vi "GIS Printer_Process.vi"(8 "error in":errorcluster, 9 "notifierSync":refnum<notifier>, 10 "TopLevel":refnum<class "TopLevel.lvclass">, 11 "GIS Printer in":refnum<class "GIS Printer.lvclass">) -> (3 "GIS Printer out":refnum<class "GIS Printer.lvclass">)   [LabVIEW 2022 SP3, in "GIS Printer.lvclass"]
uses:
  GIS Printer.lvclass
  TopLevel/TopLevel.lvclass
  Typedefs/PrinterCmdStatus--Enum.ctl
  Typedefs/Command Data.ctl
  Typedefs/API Event Data.ctl
  Typedefs/API Task State.ctl
  Typedefs/API Command Cluster.ctl
  Typedefs/API Command Enum.ctl
  Typedefs/PrinterResponse--Cluster.ctl
  Typedefs/PrinterCommand--Cluster.ctl
  Motor Controller/Motor Controller.lvclass
  AbortProcess.vi
panel:
  in  "C33":bool
  in  "I33 3":bool
  in  "I33 2":bool
  in  "I33 1":bool
  in  "A33":bool
  in  "C22":bool
  in  "A22":bool
  in  "C11":bool
  in  "A11":bool
  in  "C1":bool
  in  "A1":bool
  in  "C2":bool
  in  "A2":bool
  in  "C3":bool
  in  "A3":bool
  in  "C4":bool
  in  "A4":bool
  out "error out":errorcluster
  in  "OK":bool
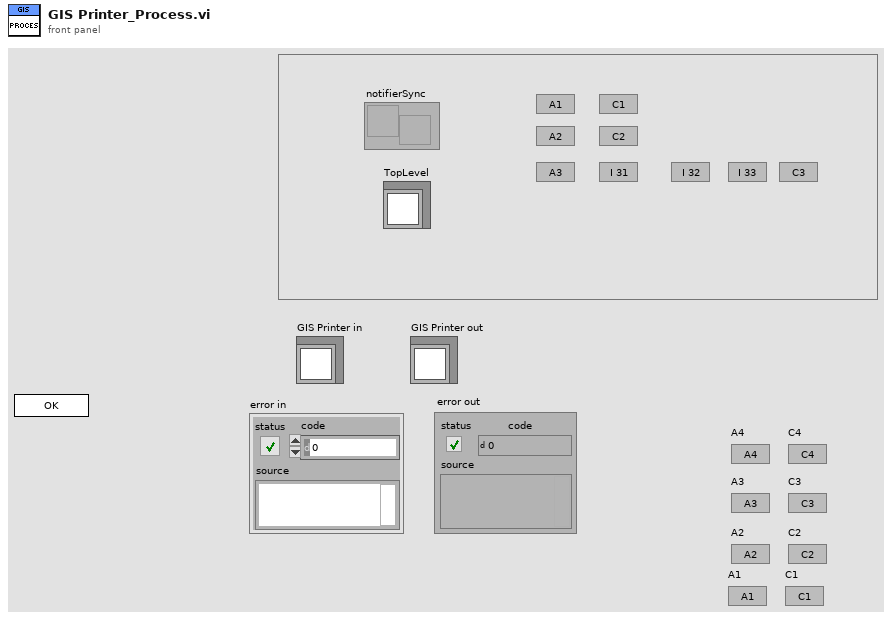
[diagram p1: front panel]
types:
  T1 = cluster{"String":string, "PrinterResponse":refnum<user-event>, "TCP":refnum<k5>, "Open":bool, "TCP 2":refnum<k5>, "Open 2":bool}
  T2 = typedef "GIS Printer.lvclass/PrinterCmdStatus--Enum.ctl" = enum16{"WaitingForAck", "Executing", "Executing Standby", "Completed", "Error"}
  T3 = typedef "GIS Printer.lvclass/Command Data.ctl" = cluster{"PrinterResponse":string, "Cmd Status":T2}
  T4 = typedef "GIS Printer.lvclass/API Event Data.ctl" = cluster{"Task":cluster{"Time Stamp":timestamp, "Timeout (ms)":u32, "Task State":T5, "Task Error":errorcluster, "Task ID":string}, "Command":variant, "Return Value":variant}
  T5 = typedef "GIS Printer.lvclass/API Task State.ctl" = enum16{"Completed", "Errored", "Pending"}
  T6 = typedef "GIS Printer.lvclass/API Command Cluster.ctl" = cluster{"Command":T7, "Arguments":string}
  T7 = typedef "GIS Printer.lvclass/API Command Enum.ctl" = enum16{"Execute Printer Command", "Abort"}
  T8 = enum32{"invalid app kind", "Development System", "Run Time System", "Student Edition", "Embedded LabVIEW", "Evaluation", "Custom"}
  T9 = typedef "GIS Printer.lvclass/PrinterCommand--Cluster.ctl" = cluster{"WaitFor":string, "SentTime":dbl, "PrinterCmdStatus":T2}
  T10 = enum32{"Invalid", "Standard", "Closed", "Hidden", "Minimized", "Maximized"}
  T11 = typedef "GIS Printer.lvclass/PrinterResponse--Cluster.ctl" = cluster{"Command":string, "Response[]":string[], "LastResponse":string, "WaitFor":string}
  T12 = cluster{"Time Stamp":timestamp, "Timeout (ms)":u32, "Task State":T5, "Task Error":errorcluster, "Task ID":string}
  T13 = typedef "GIS Printer.lvclass/PrinterConfiguration--Cluster.ctl" = cluster{"IPAddress":string, "Move Stage on RTP Command?":bool, "Stage Move Position":string, "PH1-Prime Path":path, "PH2-Prime Path":path, "PH3-Prime Path":path, "PH4-Prime Path":path, "PH5-Prime Path":path, "PH6-Prime Path":path, "PrintScriptsFolder":path, "PurgeScriptsFolder":path, "StageScriptsFolder":path, "PH1-HeatOn Path":path, "PH2-HeatOn Path":path, "PH3-HeatOn Path":path, "PH4-HeatOn Path":path, "PH5-HeatOn Path":path, "PH6-HeatOn Path":path, "PH1-HeatOff Path":path, "PH2-HeatOff Path":path, "PH3-HeatOff Path":path, "PH4-HeatOff Path":path, "PH5-HeatOff Path":path, "PH6-HeatOff Path":path}
  T14 = cluster{"Core":cluster{"Current VI Reference":refnum<vi>, "Close Panel on Exit?":bool}, "GIS Printer in":refnum<class "GIS Printer.lvclass">, "Tasks":T4[], "TO":i32, "API Executed Event":refnum<user-event>, "API Return Event":refnum<user-event>, "Task Start ms":u32, "Current Task. Return Value":variant, "TCP":refnum<k5>, "PrinterConfiguration":T13, "CmdMap":map{string, T11}, "CurrentTask":T6, "IDmap":map{string, T9}, "Motor Controller":refnum<class "Motor Controller.lvclass">, "TCP 2":refnum<k5>, "notifierSync":refnum<notifier>}
  T15 = cluster{"Current VI Reference":refnum<vi>, "Close Panel on Exit?":bool}
  T16 = typedef "TopLevel.lvclass/Digilens Config Cluster.ctl" = cluster{"Motion Controller":T17, "IO Config":T18, "PrinterConfiguration":T13, "DAQ Settings":T21}
  T17 = typedef "Motor Controller.lvclass/Motor Controller Config Data.ctl" = cluster{"Motor IP Addresss":string, "Current Position":i32, "Pulse_Per_mm":i32, "PrePrint":dbl[], "Load Position_mm":i32, "Laminate Position_mm":i32}
  T18 = typedef "IO.lvclass/IO Config Data.ctl" = cluster{"DAQDevices":T19[], "DI Channels":T20[], "DO Channels":T20[], "Material Names":string[], "AI Channels":T20[], "AO Channels":T20[]}
  T19 = typedef "IO.lvclass/DCON_DeviceConfig--Cluster.ctl" = cluster{"COM":string, "DeviceName":string, "BaudRate":u32, "Number of Channels":i32, "DeviceAddress":i32, "Enable":bool}
  T20 = typedef "IO.lvclass/Channel Data.ctl" = cluster{"Channel Name":string, "Device Name":string, "Channel No":string}
  T21 = typedef "DAQ.lvclass/TD DAQ Settings--cluster.ctl" = cluster{"Simulate DAQ":bool, "DI Settings":T22[], "AI Settings":T23[], "Relay IONames":string[], "AO IONames":string[], "AO NChan SingleTask":bool}
  T22 = typedef "DAQ.lvclass/TD DI Instrument Settings--cluster.ctl" = cluster{"Disable":bool, "DI TaskName":string, "DI RefreshIntv":i32}
  T23 = typedef "DAQ.lvclass/TD AI Instrument Settings--cluster.ctl" = cluster{"Disable":bool, "AI TaskName":string, "AI InstSettings":T24, "SimAI Ranges":T25}
  T24 = typedef "DAQ.lvclass/TD AI InstSettings--cluster.ctl" = cluster{"DaqRate":dbl, "NumSamples":i32}
  T25 = typedef "DAQ.lvclass/TD SimAI Ranges--cluster.ctl" = cluster{"lo":dbl, "hi":dbl}
  T26 = typedef "GIS Printer.lvclass/UserEvents.ctl" = cluster{"API Incoming Event":refnum<user-event>, "API Executed Event":refnum<user-event>, "API Return Event":refnum<user-event>, "Status Changed Event":refnum<user-event>, "Abort":refnum<user-event>, "stop process":refnum<user-event>, "GISPollStatus":refnum<user-event>, "GISHeadStatus":refnum<user-event>, "Error Event":refnum<user-event>}
  T27 = typedef "TopLevel.lvclass/UserEvents.ctl" = cluster{"API Incoming Event":refnum<user-event>, "API Executed Event":refnum<user-event>, "API Return Event":refnum<user-event>, "Exit Event":refnum<user-event>, "StatusChanged":refnum<user-event>, "DLP GUI Config Changed":refnum<user-event>, "AppEvent":refnum<user-event>, "Login Event":refnum<user-event>}
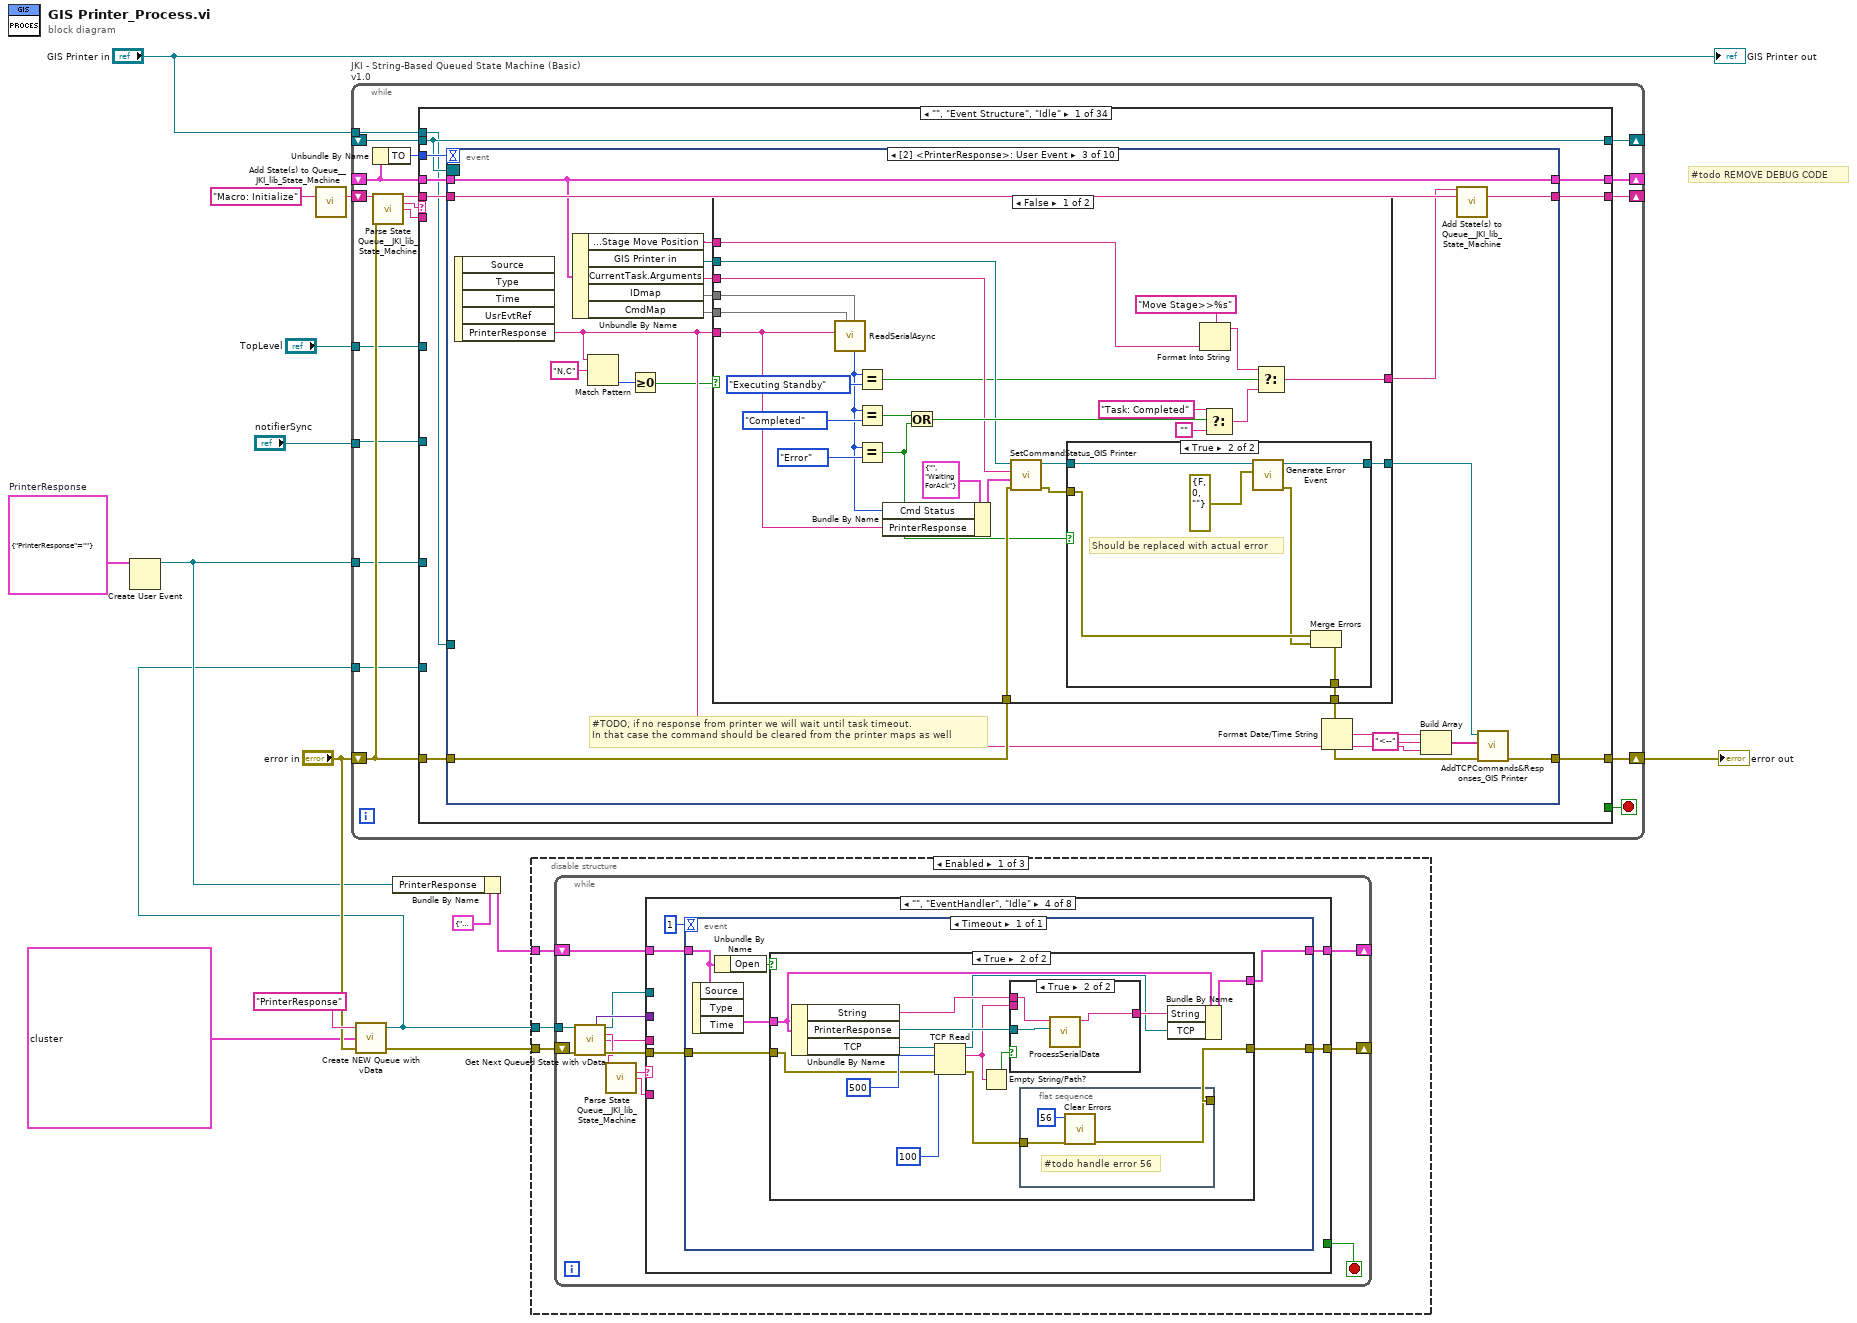
[diagram p0: block diagram]
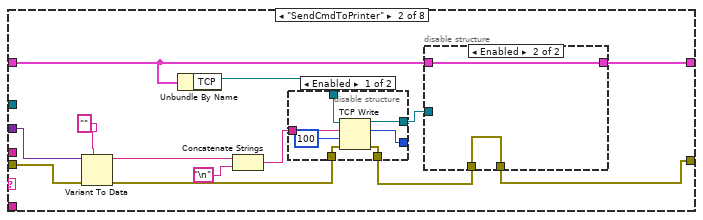
[diagram p3: hidden frame]
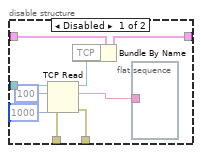
[diagram p4: hidden frame]
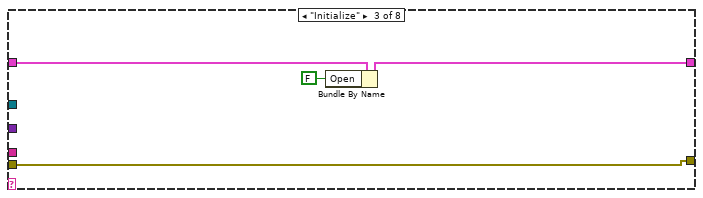
[diagram p6: hidden frame]
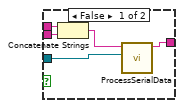
[diagram p8: hidden frame]
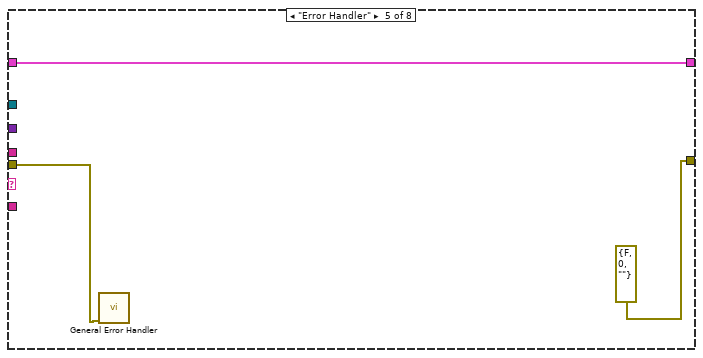
[diagram p9: hidden frame]
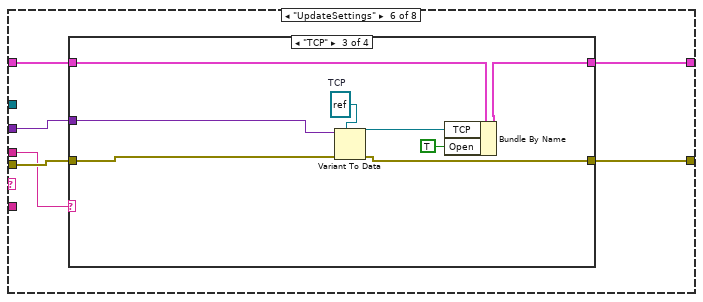
[diagram p10: hidden frame]
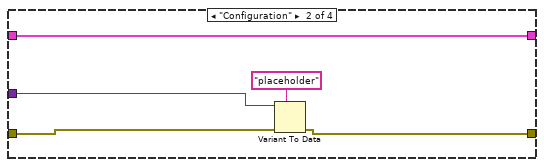
[diagram p12: hidden frame]
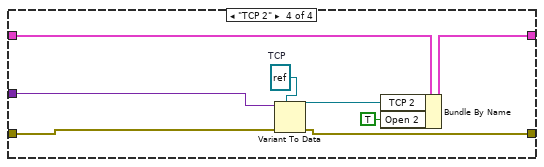
[diagram p13: hidden frame]
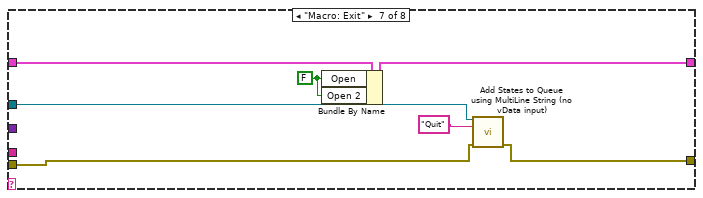
[diagram p14: hidden frame]
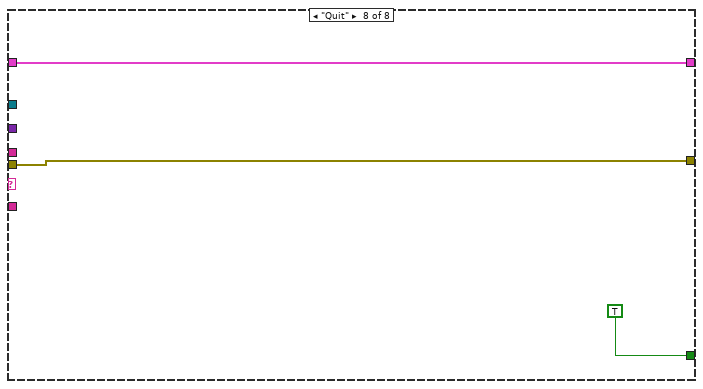
[diagram p15: hidden frame]
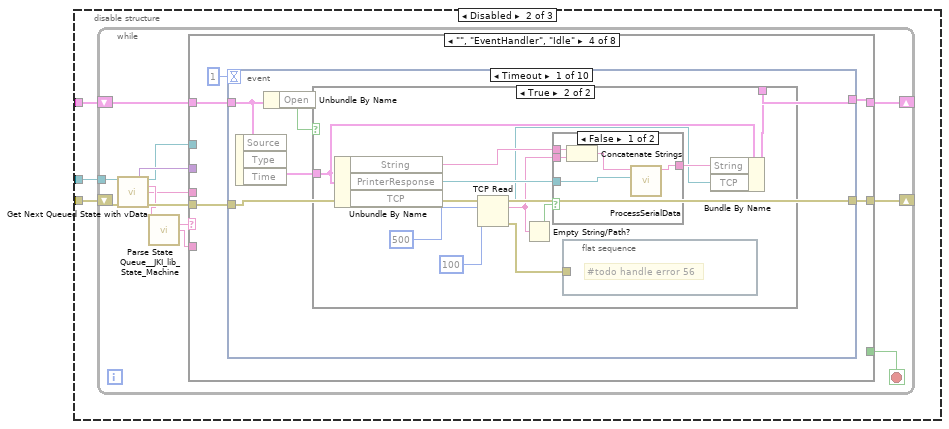
[diagram p16: hidden frame]
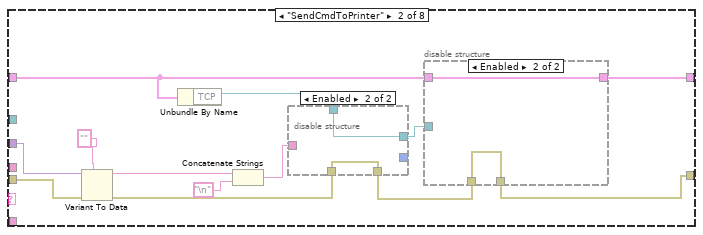
[diagram p18: hidden frame]
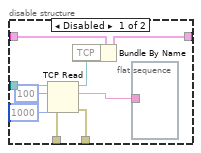
[diagram p19: hidden frame]
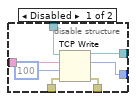
[diagram p20: hidden frame]
diagram:
  w10 = cluster{"PrinterResponse":string} {"PrinterResponse"=""}  # PrinterResponse
  # "#todo REMOVE DEBUG CODE"
  n1 = Create User Event(user event datatype=w10) -> (user event=w3:refnum<user-event>)  [unwired: 1 in, 1 out]
  n2 = call <vilib>:"Add State(s) to Queue__JKI_lib_State_Machine.vi"("State(s) in (\"\")"="Macro: Initialize") -> ("States Out"=w15:string)  [unwired: 14 in]
  n3 = call <vilib>:"Create NEW Queue with vData.vi"("error in (no error)"="error in", "Initial States"=cluster{"state":string, "vData":variant}[] [{"state"="Initialize", "vData"=variant}, {"state"="Idle", "vData"=variant}], "Name (SMQ)"="PrinterResponse") -> ("error out"=w8:errorcluster, "queue out"=w2:refnum<queue>)  [unwired: 1 in]
  n4 = while "JKI - String-Based Queued State Machine (Basic) v1.0" {
    shift-right: [w26] -> _
    shift-left: _ -> [w20]
    shift-right: [w29] -> w12
    shift-left: "error in" -> [w25]
    shift-right: [w28] -> _
    shift-left: w15 -> [w30]
    tunnel: "GIS Printer in" -> [w24]
    shift-right: [w23] -> _
    shift-left: _ -> [w22]
    tunnel: "TopLevel" -> [w19]
    tunnel: w3 -> [w18]
    tunnel: w2 -> [w17]
    tunnel: "notifierSync" -> [w16]
    stop <- w27 stop-if-true
    n5 = Unbundle By Name(w20) -> ("TO"=w21:i32)
    n6 = call <vilib>:"Parse State Queue__JKI_lib_State_Machine.vi"("State Queue"=w30, "Error In (no error)"=w25) -> ("Remaining States"=w32:string, "Current State"=w33:string, "Arguments"=w31:string)  [unwired: 11 in]
    n7 = case shown="\"\", \"Event Structure\", \"Idle\"" w33 {
      selector: w33 -> [_ _ w250 _ _ _ _ _ _ _ _ _ _ _ _ _ _ _ _ _ _ _ _ _ _ _ _ _ _ _ _ _ _ _]
      tunnel: w32 -> [w42 w248 w254 w273 w280 w286 w291 w299 w334 w341 w346 w352 w359 w371 w398 _ w417 w421 w439 w444 w446 _ w504 w519 w534 w542 w559 w570 w589 w606 w622 w642 w667 w705]
      tunnel: w31 -> [_ _ _ _ _ _ _ _ _ _ _ _ w354 w365 _ _ _ _ _ _ _ _ _ _ _ w536 _ _ _ _ _ _ _ _]
      tunnel: w20 -> [w40 w245 w252 w264 w277 w284 w288 w294 _ w336 w343 w350 w357 w367 w395 w400 w415 w419 w436 w443 w447 w454 w503 w520 w524 w541 w560 w567 w586 w605 w620 w640 w664 w702]
      tunnel: [w39 w246 w256 w270 errorcluster {"status"=FALSE, "code"=0, "source"=""} ("error out") w283 w289 w293 w326 w337 w344 w347 w355 w368 w396 w403 w406 w420 w434 w442 w445 w455 w483 w518 w525 w537 w558 w565 w584 w600 w616 w637 w672 w701] -> w29
      tunnel: w25 -> [w38 w246 w255 w270 w276 w283 w289 w292 w325 w338 w344 w348 w356 w369 w396 w403 w405 w420 w426 w441 w445 w461 w494 w518 w525 w539 w558 w568 w587 w604 w615 w636 w671 w700]
      tunnel: [w41 w247 w253 w272 w279 w285 w290 w298 w333 w340 w345 w351 w358 w370 w397 w402 w416 w421 w438 w444 w446 w467 w504 w519 w534 w542 w559 w570 w589 w606 w622 w642 w668 w706] -> w28
      tunnel: [_ _ _ _ _ TRUE _ _ _ _ _ _ _ _ _ _ _ _ _ _ _ _ _ _ _ _ _ _ _ _ _ _ _ _] -> w27
      tunnel: [w37 w245 w252 w271 w277 w284 w288 w294 w332 w336 w343 w350 w357 w367 w395 w400 w415 w419 w436 w443 w447 w459 w499 w520 w524 w541 w560 w569 w588 w605 w620 w640 w665 w699] -> w26
      tunnel: w21 -> [w36 _ _ _ _ _ _ _ _ _ _ _ _ _ _ _ _ _ _ _ _ _ _ _ _ _ _ _ _ _ _ _ _ _]
      tunnel: w24 -> [w34 _ _ _ _ _ _ _ w327 _ _ _ _ _ _ _ _ _ _ _ _ _ _ _ _ _ _ _ _ _ _ w632 w663 _]
      tunnel: [w35 w244 w249 w261 w274 w281 w287 w297 w330 w335 w342 w349 w353 w364 w394 w399 w408 w418 w437 w440 w448 w468 w505 w521 w535 w543 w561 w571 w590 w607 w621 w641 w675 w707] -> w23
      tunnel: w22 -> [w35 w244 w249 w261 w274 w281 w287 w297 w330 w335 w342 w349 w353 w364 w394 w399 w408 w418 _ w440 w448 w468 w505 w521 w535 w543 w561 w571 w590 w607 w621 w641 w675 w707]
      tunnel: w19 -> [_ _ _ _ _ _ _ _ w318 _ _ _ _ _ _ _ _ _ w429 _ _ _ _ _ w522 _ _ _ _ _ _ _ _ _]
      tunnel: w18 -> [_ _ _ _ _ _ _ _ _ _ _ _ _ _ _ _ _ _ w425 _ _ _ _ _ _ _ _ _ _ _ _ _ _ _]
      tunnel: w17 -> [_ _ _ _ _ _ _ _ _ _ _ _ _ _ _ _ w404 _ _ _ _ _ w477 _ _ _ _ w564 w583 _ _ _ _ _]
      tunnel: w16 -> [_ _ _ _ _ _ _ _ w300 _ _ _ _ _ _ _ _ _ _ _ _ _ _ _ _ _ _ _ _ _ _ _ _ _]
      frame "", "Event Structure", "Idle" {
        n8 = event shown="[2] <PrinterResponse>: User Event" {
          selector: w35 -> [_ _ _ _ _ _ _ _ _ _]
          dyn-events: _ -> [_ _ _ _ _ _ _ _ _ _]
          timeout: w36 -> [_ _ _ _ _ _ _ _ _ _]
          tunnel: w42 -> [w51 w56 w76 w119 w124 w132 w138 w142 w150 w227]
          tunnel: [w50 w55 w75 w118 w123 w131 w137 w141 w151 w228] -> w41
          tunnel: w40 -> [w48 w53 w74 w116 w121 w126 w135 w139 w154 w226]
          tunnel: [w49 w54 w63 w117 w122 w130 w136 w140 w153 w220] -> w39
          tunnel: w38 -> [w49 w54 w68 w117 w122 w130 w136 w140 w152 w221]
          tunnel: [w48 w53 w74 w116 w121 w127 w135 w139 w155 w223] -> w37
          tunnel: w34 -> [_ _ _ _ _ _ _ _ w143 _]
          event Timeout {
            n9 = event-data() -> ()  [unwired: 1 in, 1 out]
            n10 = Unbundle By Name(w48) -> ("Tasks"=w47:T4[])
            n11 = Empty Array?(array=w47) -> (empty?=w46:bool)
            n12 = Select(t="", s=w46, f="Task: Check Timeout") -> (s? t:f=w43:string)
            n13 = call <vilib>:"Add State(s) to Queue__JKI_lib_State_Machine.vi"("State(s) in Front (\"\")"=w43, "State(s) in (\"\")"=w51) -> ("States Out"=w50:string)  [unwired: 13 in]
          }
          event User Event {
            n14 = event-data() -> ()  [unwired: 1 in, 5 out]
            n15 = call <vilib>:"Add State(s) to Queue__JKI_lib_State_Machine.vi"("State(s) in Front (\"\")"="API: Abort" ("State(s) in Front (\"\")"), "State(s) in (\"\")"=w56) -> ("States Out"=w55:string)  [unwired: 13 in]
          }
          event User Event {
            # "#TODO, if no response from printer we will wait until task timeout.\nIn that case the command should be cleared from the printer maps as well"
            n16 = event-data() -> ("PrinterResponse"=w61:string)  [unwired: 1 in, 4 out]
            n17 = Unbundle By Name(w74) -> ("PrinterConfiguration.Stage Move Position"=w57:string, "GIS Printer in"=w70:refnum<class "GIS Printer.lvclass">, "CurrentTask.Arguments"=w69:string, "IDmap"=w73:map{string, T9}, "CmdMap"=w72:map{string, T11})
            n18 = Match Pattern(string=w61, regular expression="N,C") -> (offset past match=w59:i32)  [unwired: 1 in, 3 out]
            n19 = Greater Or Equal To 0?(x=w59) -> (x >= 0?=w58:bool)
            n20 = case shown="False" w58 {
              tunnel: w73 -> [w103 _]
              tunnel: w72 -> [w102 _]
              tunnel: [w85 ""] -> w71
              tunnel: w70 -> [w95 w113]
              tunnel: w69 -> [w94 _]
              tunnel: w68 -> [w91 w114]
              tunnel: [w77 w113] -> w65
              tunnel: [w79 w114] -> w64
              tunnel: w61 -> [w90 _]
              tunnel: w57 -> [w84 _]
              frame False {
                n21 = call "ReadSerialAsync.vi"("IDmap"=w103, "CmdMap"=w102, "input Str"=w90) -> ("PrinterCmdStatus"=w88:T2)  [unwired: 5 in, 3 out]
                n22 = Equal?(x=w88, y=PrinterCmdStatus--Enum."Executing Standby") -> (x = y?=w87:bool)
                n23 = Equal?(x=w88, y=PrinterCmdStatus--Enum."Completed") -> (x = y?=w100:bool)
                n24 = Equal?(x=w88, y=PrinterCmdStatus--Enum."Error") -> (x = y?=w81:bool)
                n25 = Bundle By Name(cluster=T3 {"PrinterResponse"="", "Cmd Status"=enum."WaitingForAck"} ("Command Data"), "Cmd Status"=w88, "PrinterResponse"=w90) -> (w92:T3)
                n26 = Or(x=w100, y=w81) -> (x .or. y?=w98:bool)
                n27 = call-dynamic "SetCommandStatus_GIS Printer.vi"("error in (no error)"=w91, "Command Data"=w92, "Command"=w94, "GIS Printer In"=w95) -> ("error out"=w80:errorcluster, "GIS Printer Out"=w78:refnum<class "GIS Printer.lvclass">)  [unwired: 6 in]
                n28 = case shown="True" w81 {
                  tunnel: w80 -> [w105 w108]
                  tunnel: [w105 w107] -> w79
                  tunnel: w78 -> [w104 w110]
                  tunnel: [w104 w109] -> w77
                  frame False {
                  }
                  frame True {
                    # "Should be replaced with actual error"
                    n29 = call-dynamic "Generate Error Event.vi"("Error"=errorcluster {"status"=FALSE, "code"=0, "source"=""}, "GIS Printer in"=w110) -> ("error out"=w106:errorcluster, "GIS Printer out"=w109:refnum<class "GIS Printer.lvclass">)  [unwired: 8 in]
                    n30 = Merge Errors(w108, w106) -> (w107:errorcluster)
                  }
                }
                n31 = Format Into String(format string="Move Stage>>%s" ("t"), w84) -> (resulting string=w82:string)  [unwired: 2 in, 1 out]
                n32 = Select(t="Task: Completed", s=w98, f="") -> (s? t:f=w86:string)
                n33 = Select(t=w82, s=w87, f=w86) -> (s? t:f=w85:string)
              }
              frame True {
                # "NC means good connection\nNZ is bad"
              }
            }
            n34 = Format Date/Time String() -> (date/time string=w67:string)  [unwired: 3 in]
            n35 = Build Array(w67, "<--", w61) -> (w62:string[])
            n36 = call <vilib>:"Add State(s) to Queue__JKI_lib_State_Machine.vi"("State(s) in Front (\"\")"=w71, "State(s) in (\"\")"=w76) -> ("States Out"=w75:string)  [unwired: 13 in]
            n37 = call-dynamic "AddTCPCommands&Responses_GIS Printer.vi"("error in (no error)"=w64, "Command \\ Response"=w62, "GIS Printer In"=w65) -> ("error out"=w63:errorcluster)  [unwired: 7 in, 1 out]
          }
          event "OK": Value Change {
            # "Exit Button Value Change (pressed) Event\n(this executes Macro: Exit to terminate the VI)"
            n38 = event-data() -> ()  [unwired: 1 in, 1 out]
            n39 = call <vilib>:"Add State(s) to Queue__JKI_lib_State_Machine.vi"("State(s) in Front (\"\")"="Macro: Exit", "State(s) in (\"\")"=w119) -> ("States Out"=w118:string)  [unwired: 13 in]
          }
          event User Event {
            # "Exit Button Value Change (pressed) Event\n(this executes Macro: Exit to terminate the VI)"
            n40 = event-data() -> ()  [unwired: 1 in, 5 out]
            n41 = disable-structure shown="Disabled" {
              disable-tunnel: ["Macro: Exit" _] -> w120
              frame Disabled {
              }
              frame Enabled {
              }
            }
            n42 = call <vilib>:"Add State(s) to Queue__JKI_lib_State_Machine.vi"("State(s) in Front (\"\")"=w120, "State(s) in (\"\")"=w124) -> ("States Out"=w123:string)  [unwired: 13 in]
          }
          event User Event {
            n43 = event-data() -> ("Command"=w129:string, "Data"=w128:variant)  [unwired: 1 in, 4 out]
            n44 = case shown="Default" w129 {
              tunnel: w128 -> [_]
              tunnel: w126 -> [w133]
              tunnel: [w133] -> w127
              frame Default {
              }
            }
            n45 = call <vilib>:"Add State(s) to Queue__JKI_lib_State_Machine.vi"("State(s) in (\"\")"=w132) -> ("States Out"=w131:string)  [unwired: 14 in]
          }
          event User Event {
            # "Exit Button Value Change (pressed) Event\n(this executes Macro: Exit to terminate the VI)"
            n46 = event-data() -> ()  [unwired: 1 in, 5 out]
            n47 = call <vilib>:"Add State(s) to Queue__JKI_lib_State_Machine.vi"("State(s) in Front (\"\")"="Macro: Exit", "State(s) in (\"\")"=w138) -> ("States Out"=w137:string)  [unwired: 13 in]
          }
          event Panel Close? {
            # "Close Panel button (pressed) Event\n(this executes Macro: Exit to terminate the VI)"
            n48 = event-data() -> ()  [unwired: 1 in, 1 out]
            n49 = event-data() -> ()  [unwired: 2 in, 1 out]
            n50 = call <vilib>:"Add State(s) to Queue__JKI_lib_State_Machine.vi"("State(s) in (\"\")"=w142) -> ("States Out"=w141:string)  [unwired: 14 in]
          }
          event User Event {
            n51 = event-data() -> ("Task"=w158:T12, "Command"=w157:variant)  [unwired: 1 in, 4 out]
            n52 = Bundle By Name(cluster=T4 {"Task"={"Time Stamp"=timestamp(0 s since 1904-01-01), "Timeout (ms)"=0, "Task State"=enum."Completed", "Task Error"={"status"=FALSE, "code"=0, "source"=""}, "Task ID"=""}, "Command"=variant, "Return Value"=variant} ("API Event Data"), "Task"=w158, "Command"=w157) -> (w148:T4)
            n53 = Unbundle By Name(w154) -> ("Tasks"=w156:T4[])
            n54 = Unbundle By Name(w148) -> ("Task.Task ID"=w147:string)
            n55 = Empty Array?(array=w156) -> (empty?=w145:bool)
            n56 = Equal?(x=w147, y="AbortPrint") -> (x = y?=w144:bool)
            n57 = case shown="True" w144 {
              tunnel: w156 -> [w168 _]
              tunnel: [w167 w207] -> w155
              tunnel: w154 -> [w166 w207]
              tunnel: [w165 w196] -> w153
              tunnel: w152 -> [w164 w198]
              tunnel: [w163 w199] -> w149
              tunnel: w148 -> [w162 w200]
              tunnel: w145 -> [w161 _]
              tunnel: w143 -> [w160 _]
              frame False {
                n58 = case shown="True" w161 {
                  tunnel: w168 -> [w189 w195]
                  tunnel: w162 -> [w188 w194]
                  tunnel: w166 -> [w187 w193]
                  tunnel: [w185 w191] -> w167
                  tunnel: w162 -> [w184 _]
                  tunnel: w164 -> [w169 w190]
                  tunnel: [w180 w190] -> w165
                  tunnel: [w177 _] -> w163
                  tunnel: w160 -> [w172 _]
                  frame True {
                    n59 = Unbundle By Name(w184) -> ("Command"=w183:variant)
                    n60 = call-dynamic "SetPrinterBusy_Status_GIS Printer.vi"("error in (no error)"=w169, "Printer Busy?"=TRUE, "GIS Printer In"=w172) -> ("error out"=w170:errorcluster)  [unwired: 7 in, 1 out]
                    n61 = Build Array (concatenate)(w189, w188) -> (w186:T4[])
                    n62 = Variant To Data(error in=w170, type=T6 {"Command"=enum."Execute Printer Command", "Arguments"=""} ("API Command Cluster"), Variant=w183) -> (data=w173:T6, error out=w181:errorcluster)
                    n63 = Tick Count (ms)() -> (millisecond timer value=w175:u32)
                    n64 = Unbundle By Name(w173) -> ("Command"=w178:T7, "Arguments"=w176:string)
                    n65 = Bundle By Name(cluster=w187, "TO"=100, "Tasks"=w186, "Task Start ms"=w175, "CurrentTask"=w173) -> (w185:T14)
                    n66 = Format Into String(format string="API: %s>>%s", error in=w181, w178, w176) -> (resulting string=w177:string, error out=w180:errorcluster)  [unwired: 1 in]
                  }
                  frame False {
                    n67 = Build Array (concatenate)(w195, w194) -> (w192:T4[])
                    n68 = Bundle By Name(cluster=w193, "Tasks"=w192) -> (w191:T14)
                  }
                }
              }
              frame True {
                # "Abort should not send a task complete"
                n69 = Unbundle By Name(w200) -> ("Command"=w206:variant)
                n70 = Variant To Data(error in=w198, type=T6 {"Command"=enum."Execute Printer Command", "Arguments"=""} ("API Command Cluster"), Variant=w206) -> (data=w201:T6, error out=w197:errorcluster)
                n71 = Unbundle By Name(w201) -> ("Command"=w203:T7, "Arguments"=w202:string)
                n72 = Format Into String(format string="API: %s>>%s", error in=w197, w203, w202) -> (resulting string=w199:string, error out=w196:errorcluster)  [unwired: 1 in]
              }
            }
            n73 = call <vilib>:"Add State(s) to Queue__JKI_lib_State_Machine.vi"("State(s) in Front (\"\")"=w149, "State(s) in (\"\")"=w150) -> ("States Out"=w151:string)  [unwired: 13 in]
          }
          event User Event {
            n74 = event-data() -> ("Task"=w214:T12, "Command"=w218:variant, "Return Value"=w217:variant)  [unwired: 1 in, 4 out]
            n75 = Unbundle By Name(w226) -> ("API Return Event"=w211:refnum<user-event>, "Tasks"=w225:T4[])
            n76 = Bundle By Name(cluster=T4 {"Task"={"Time Stamp"=timestamp(0 s since 1904-01-01), "Timeout (ms)"=0, "Task State"=enum."Completed", "Task Error"={"status"=FALSE, "code"=0, "source"=""}, "Task ID"=""}, "Command"=variant, "Return Value"=variant} ("API Event Data"), "Task"=w214, "Command"=w218, "Return Value"=w217) -> (w216:T4)
            n77 = Delete From Array(array=w225, index=0) -> (deleted portion=w215:T4, array with subset deleted=w222:T4[])  [unwired: 1 in]
            n78 = Unbundle By Name(w215) -> ("Task.Task ID"=w213:string)
            n79 = Unbundle By Name(w214) -> ("Task ID"=w212:string, "Task State"=w209:T5)
            n80 = Equal?(x=w213, y=w212) -> (x = y?=w210:bool)
            n81 = case shown="True" w210 {
              tunnel: w226 -> [w230 w243]
              tunnel: [w230 w242] -> w223
              tunnel: w222 -> [_ w241]
              tunnel: w211 -> [_ w240]
              tunnel: w221 -> [w229 w237]
              tunnel: [w229 w238] -> w220
              tunnel: w216 -> [_ w239]
              tunnel: w209 -> [_ w236]
              tunnel: [_ w231] -> w208
              frame False {
              }
              frame True {
                n82 = Equal?(x=w236, y=API_Task_State."Errored") -> (x = y?=w234:bool)
                n83 = Select(t="Task: Remove on Error", s=w234, f="Task: Check Pending") -> (s? t:f=w231:string)
                n84 = Bundle By Name(cluster=w243, "Tasks"=w241) -> (w242:T14)
                n85 = Generate User Event(user event=w240, event data cluster=w239, error in=w237) -> (error out=w238:errorcluster)  [unwired: 1 in, 1 out]
              }
            }
            n86 = call <vilib>:"Add State(s) to Queue__JKI_lib_State_Machine.vi"("State(s) in Front (\"\")"=w208, "State(s) in (\"\")"=w227) -> ("States Out"=w228:string)  [unwired: 13 in]
          }
        }
      }
      frame "---------- Core ----------" {
        n87 = call <vilib>:"Add State(s) to Queue__JKI_lib_State_Machine.vi"("State(s) in (\"\")"=w248) -> ("States Out"=w247:string)  [unwired: 14 in]
      }
      frame Default {
        w259 = 42 items=["No error", "Argument error", "Memory is full", "Out of zone", "End of file", "File already open", "Generic file I/O error", "File not found", "File permission error", "Disk is full", "Duplicate path", "Too many files open", "System feature not enabled", "Resource file not found", "Cannot add resource", "Resource not found", "Image not found", "Image memory error", "Pen does not exist", "Config type invalid", "Config token not found", "Config parse error", "Config memory error", "Bad external code format", "Bad external code offset", "External code not present", "Null window", "Destroy window error", "Null menu", "Print aborted", "Bad print record", "Print driver error", "Windows error during printing", "Memory error during printing", "Print dialog error", "Generic print error", "Invalid device refnum", "Device not found", "Device parameter error", "Device unit error", "Cannot open device", "Device call aborted", "Generic error", "Cancelled by user", "Object ID too low", "Object ID too high", "Object not in heap", "Unknown heap", "Unknown object (invalid DefProc)", "Unknown object (DefProc not in table)", "Message out of range", "Invalid (null) method", "Unknown message", "Manager call not supported", "Bad address", "Network operation in progress", "Network operation timed out", "Connection is busy", "Network attribute not supported", "Network error", "Address in use", "System out of memory", "Connection aborted", "Connection refused", "Not connected", "Already connected", "Connection closed", "Initialization error (interapplication manager)", "Bad occurrence", "Wait on unbound occurrence handler", "Occurrence queue overflow", "Datalog type conflict", "Unused", "Unrecognized type (interapplication manager)", "Memory corrupt", "Failed to make temporary DLL", "Old CIN version", "Drag socket not found", "Failed to load drop-object", "Failed to register OLE object", "Failed to release OLE object", "Format specifier type mismatch", "Unknown format specifier", "Too few format specifiers", "Too many format specifiers", "Scan failed", "Newer CIN version", "Error converting to variant", "Runtime menu error", "Password tampered", "Variant attribute not found", "Incompatible variant data type", "Event data is not available", "Event Store is not present", "Occurrence is not found", "Event Queue is not created", "Event info is not available", "Refnum passed is NULL", "Error retrieving Class GUID", "Error retrieving CoClass GUID", "Error retrieving TypeLib GUID.", "Bad built application magic bytes.", "Specific driver is different from the specific driver associated with the Logical Name.", "There is no session opened to the class driver.", "Max Error", "MAX - Error with config objects", "MAX - Error loading configuration", "MAX - Group not supported"]
        # "Current State"
        # "Handle mistyped state name (developer tool)"
        n88 = Format Into String(format string="Software Exception: Unhandled State \"%s\"." ("message"), error in=w255, w250) -> (resulting string=w258:string, error out=w257:errorcluster)  [unwired: 1 in]
        n89 = call <vilib>:"Error Cluster From Error Code.vi"("show call chain? (False)"=TRUE, "error in (no error)"=w257, "error message (\"\")"=w258, "error code (0)"=w259) -> ("error out"=w256:errorcluster)  [unwired: 5 in]
        n90 = call <vilib>:"Add State(s) to Queue__JKI_lib_State_Machine.vi"("State(s) in (\"\")"=w254) -> ("States Out"=w253:string)  [unwired: 14 in]
      }
      frame "Initialize Core Data" {
        # "originally closed?"
        # "exe?"
        # "If panel starts closed or is an EXE, then close it when we exit"
        n91 = property class="VI"() -> ("Front Panel.Open"=w269:bool)  [unwired: 2 in, 2 out]
        n92 = property class="App"() -> ("App.Kind"=w268:T8)  [unwired: 2 in, 2 out]
        n93 = control-ref of="Current VI Reference"() -> (w262:refnum<vi>)
        n94 = Not(x=w269) -> (.not. x?=w266:bool)
        n95 = Equal?(x=w268, y=T8."Run Time System" ("Application:Kind")) -> (x = y?=w265:bool)
        n96 = Or(x=w266, y=w265) -> (x .or. y?=w263:bool)
        n97 = Bundle By Name(cluster=w264, "Core.Current VI Reference"=w262, "Core.Close Panel on Exit?"=w263) -> (w271:T14)
        n98 = call <vilib>:"Add State(s) to Queue__JKI_lib_State_Machine.vi"("State(s) in (\"\")"=w273) -> ("States Out"=w272:string)  [unwired: 14 in]
      }
      frame "Error Handler" {
        # "Unhandled Error -- Display it"
        # "Clear error"
        n99 = call <vilib>:"General Error Handler.vi"("error in (no error)"=w276) -> ()  [unwired: 10 in, 5 out]
        n100 = call <vilib>:"Add State(s) to Queue__JKI_lib_State_Machine.vi"("State(s) in Front (\"\")"="/* Post Error States", "State(s) in (\"\")"=w280) -> ("States Out"=w279:string)  [unwired: 13 in]
      }
      frame "Exit" {
        n101 = call <vilib>:"Add State(s) to Queue__JKI_lib_State_Machine.vi"("State(s) in (\"\")"=w286) -> ("States Out"=w285:string)  [unwired: 14 in]
      }
      frame "---------- Data ----------" {
        n102 = call <vilib>:"Add State(s) to Queue__JKI_lib_State_Machine.vi"("State(s) in (\"\")"=w291) -> ("States Out"=w290:string)  [unwired: 14 in]
      }
      frame "Process: Sync" {
        n103 = Unbundle By Name(w294) -> ("notifierSync"=w296:refnum<notifier>)
        n104 = Send Notification(notification=TRUE, notifier=w296, error in (no error)=w292) -> (error out=w293:errorcluster)  [unwired: 1 out]
        n105 = call <vilib>:"Add State(s) to Queue__JKI_lib_State_Machine.vi"("State(s) in (\"\")"=w299) -> ("States Out"=w298:string)  [unwired: 14 in]
      }
      frame "Data: Initialize" {
        w301 = refnum<k5> refnum  # TCP 2
        w304 = refnum<class "Motor Controller.lvclass"> refnum  # Motor Controller
        w305 = map{string, T9} {}  # IDmap
        w310 = map{string, T11} {}  # CmdMap
        w311 = T11 {"Command"="", "Response[]"=[], "LastResponse"="", "WaitFor"=""}  # Response
        w312 = T6 {"Command"=enum."Execute Printer Command", "Arguments"=""}  # CurrentTask
        w319 = refnum<k5> refnum  # TCP
        w320 = variant  # Current Task. Return Value
        w322 = u32 0  # Task Start ms
        w328 = 100  # TO
        w329 = T4[] []  # Tasks
        w331 = T15 {"Current VI Reference"=refnum, "Close Panel on Exit?"=FALSE}  # Core
        n106 = property class="TopLevel.lvclass"(reference=w318) -> ("Methods:Accessors:Digilens Config"=w317:T16, "Methods:Accessors:Motor Controller"=w303:refnum<class "Motor Controller.lvclass">)  [unwired: 1 in, 2 out]
        n107 = Unbundle By Name(w317) -> ("PrinterConfiguration"=w316:T13)
        n108 = Coerce To Type(0:w303, 1:w304) -> (2:w302:refnum<class "Motor Controller.lvclass">)
        n109 = node("Commands" ("key"), T9 {"WaitFor"="", "SentTime"=0.0, "PrinterCmdStatus"=enum."WaitingForAck"} ("Cluster")) -> (w308:map{string, T9})
        n110 = Coerce To Type(0:w308, 1:w305) -> (2:w307:map{string, T9})
        n111 = call-dynamic "GetEvents_GIS Printer.vi"("error in (no error)"=w325, "TopLevel in"=w327) -> ("error out"=w326:errorcluster, "UserEvents"=w324:T26)  [unwired: 7 in, 1 out]
        n112 = Unbundle By Name(w324) -> ("API Executed Event"=w323:refnum<user-event>, "API Return Event"=w321:refnum<user-event>)
        n113 = node("CmdID" ("key"), w311) -> (w314:map{string, T11})
        n114 = Coerce To Type(0:w314, 1:w310) -> (2:w313:map{string, T11})
        n115 = call <vilib>:"Add State(s) to Queue__JKI_lib_State_Machine.vi"("State(s) in (\"\")"=w334) -> ("States Out"=w333:string)  [unwired: 14 in]
        n116 = Bundle("Core"=w331, "GIS Printer in"=w327, "Tasks"=w329, "TO"=w328, "API Executed Event"=w323, "API Return Event"=w321, "Task Start ms"=w322, "Current Task. Return Value"=w320, "TCP"=w319, "PrinterConfiguration"=w316, "CmdMap"=w313, "CurrentTask"=w312, "IDmap"=w307, "Motor Controller"=w302, "TCP 2"=w301, "notifierSync"=w300) -> (w332:T14)  [unwired: 1 in]
      }
      frame "Data: Cleanup" {
        n117 = Unbundle By Name(w336) -> ("Core.Current VI Reference"=w339:refnum<vi>)
        n118 = Close Reference(reference=w339, error in (no error)=w338) -> (error out=w337:errorcluster)
        n119 = call <vilib>:"Add State(s) to Queue__JKI_lib_State_Machine.vi"("State(s) in (\"\")"=w341) -> ("States Out"=w340:string)  [unwired: 14 in]
      }
      frame "---------- UI ----------" {
        n120 = call <vilib>:"Add State(s) to Queue__JKI_lib_State_Machine.vi"("State(s) in (\"\")"=w346) -> ("States Out"=w345:string)  [unwired: 14 in]
      }
      frame "UI: Initialize" {
        n121 = call <userlib>:"Fit VI window to Largest Dec__ogtk.vi"("error in (no error)"=w348) -> ("error out"=w347:errorcluster)  [unwired: 5 in, 1 out]
        n122 = call <vilib>:"Add State(s) to Queue__JKI_lib_State_Machine.vi"("State(s) in (\"\")"=w352) -> ("States Out"=w351:string)  [unwired: 14 in]
      }
      frame "UI: Cursor Set" {
        # "Argument"
        n123 = case shown="\"Idle\", Default" w354 {
          tunnel: w356 -> [w361 w363]
          tunnel: [w360 w362] -> w355
          frame "Idle", Default {
            n124 = call <vilib>:"Unset Busy.vi"("error in (no error)"=w361) -> ("error out"=w360:errorcluster)  [unwired: 10 in]
          }
          frame "Busy" {
            n125 = call <vilib>:"Set Busy.vi"("error in (no error)"=w363) -> ("error out"=w362:errorcluster)  [unwired: 9 in, 1 out]
          }
        }
        n126 = call <vilib>:"Add State(s) to Queue__JKI_lib_State_Machine.vi"("State(s) in (\"\")"=w359) -> ("States Out"=w358:string)  [unwired: 14 in]
      }
      frame "UI: Front Panel State" {
        # "Argument"
        n127 = Unbundle By Name(w367) -> ("Core.Current VI Reference"=w366:refnum<vi>)
        n128 = case shown="\"Open\", Default" w365 {
          tunnel: w369 -> [w375 w388]
          tunnel: [w377 w389] -> w368
          tunnel: w366 -> [w376 w386]
          frame "Open", Default {
            n129 = property class="VI"(reference=w376, error in=w375) -> (reference out=w373:refnum<vi>, error out=w374:errorcluster, "Front Panel.Open"=w372:bool)
            n130 = case shown="False" w372 {
              tunnel: [w380 w383] -> w377
              tunnel: w374 -> [w379 w383]
              tunnel: w373 -> [w378 _]
              frame False {
                n131 = invoke class="VI" method="FP.Open"(reference=w378, error in=w379, "Activate"=TRUE, "State"=T10."Standard") -> (error out=w380:errorcluster)  [unwired: 1 in, 4 out]
              }
              frame True {
              }
            }
          }
          frame "Close" {
            n132 = property class="VI"(reference=w386, error in=w388) -> (reference out=w385:refnum<vi>, error out=w387:errorcluster, "Front Panel.Open"=w384:bool)
            n133 = case shown="True" w384 {
              tunnel: [w390 w393] -> w389
              tunnel: w387 -> [w390 w392]
              tunnel: w385 -> [_ w391]
              frame False {
              }
              frame True {
                n134 = invoke class="VI" method="FP.Close"(reference=w391, error in=w392) -> (error out=w393:errorcluster)  [unwired: 1 in, 2 out]
              }
            }
          }
        }
        n135 = call <vilib>:"Add State(s) to Queue__JKI_lib_State_Machine.vi"("State(s) in (\"\")"=w371) -> ("States Out"=w370:string)  [unwired: 14 in]
      }
      frame "---------- Macro ----------" {
        n136 = call <vilib>:"Add State(s) to Queue__JKI_lib_State_Machine.vi"("State(s) in (\"\")"=w398) -> ("States Out"=w397:string)  [unwired: 14 in]
      }
      frame "Macro: Initialize" {
        w401 = "Data: Initialize\nInitialize Core Data\nUI: Initialize\nAction: Open Connection\nAction: Open Connection 2\n/*Action: Launch Abort Process\nEvents: Register Events\nProcess: Sync\n/*UI: Front Panel State >> Open"  # Data: Initialize Initialize Core Data UI: Initialize Action: Open Connection Action: Open Connection 2 /*Action: Launch Abort Process Events: Register Events Process: Sync /*UI: Front Panel State >> Open
        n137 = call <vilib>:"Add State(s) to Queue__JKI_lib_State_Machine.vi"("State(s) in (\"\")"=w401) -> ("States Out"=w402:string)  [unwired: 14 in]
      }
      frame "Macro: Exit" {
        n138 = call <vilib>:"Add States to Queue using MultiLine String (no vData input).vi"("queue in"=w404, "states in"="Macro: Exit", "error in"=w405) -> ("error out"=w406:errorcluster)  [unwired: 10 in, 2 out]
        n139 = Unbundle By Name(w415) -> ("Core.Close Panel on Exit?"=w414:bool)
        n140 = Select(t="UI: Front Panel State >> Close", s=w414, f="") -> (s? t:f=w411:string)
        n141 = call <vilib>:"Add State(s) to Queue__JKI_lib_State_Machine.vi"("State(s) in (\"\")"=w411, "State(s) at Back (\"\")"="Data: Cleanup\nEvents: Unregister Events\nAction: Close Connection\nExit") -> ("States Out"=w409:string)  [unwired: 13 in]
        n142 = call <vilib>:"Add State(s) to Queue__JKI_lib_State_Machine.vi"("State(s) in Front (\"\")"=w409, "State(s) in (\"\")"=w417) -> ("States Out"=w416:string)  [unwired: 13 in]
      }
      frame "---------- Events ----------" {
      }
      frame "Events: Register Events" {
        n143 = call-dynamic "GetEvents_TopLevel.vi"("error in (no error)"=w426, "TopLevel in"=w429) -> ("error out"=w427:errorcluster, "UserEvents"=w430:T27)  [unwired: 7 in, 1 out]
        n144 = Unbundle By Name(w430) -> ("Exit Event"=w428:refnum<user-event>, "AppEvent"=w422:refnum<user-event>)
        n145 = Unbundle By Name(w436) -> ("GIS Printer in"=w435:refnum<class "GIS Printer.lvclass">)
        n146 = call-dynamic "GetEvents_GIS Printer.vi"("error in (no error)"=w427, "TopLevel in"=w435) -> ("error out"=w434:errorcluster, "UserEvents"=w433:T26)  [unwired: 7 in, 1 out]
        n147 = Unbundle By Name(w433) -> ("API Incoming Event"=w432:refnum<user-event>, "API Executed Event"=w431:refnum<user-event>, "Abort"=w424:refnum<user-event>, "stop process"=w423:refnum<user-event>)
        n148 = register-events(w432, w431, w428, w425, w424, w423, w422) -> (reference out=w437:refnum<event-registration>)  [unwired: 2 in, 1 out]
        n149 = call <vilib>:"Add State(s) to Queue__JKI_lib_State_Machine.vi"("State(s) in (\"\")"=w439) -> ("States Out"=w438:string)  [unwired: 14 in]
      }
      frame "Events: Unregister Events" {
        n150 = Unregister For Events(event registration refnum=w440, error in=w441) -> (error out=w442:errorcluster)
      }
      frame "---------- API ----------" {
      }
      frame "API: Abort" {
        n151 = Unbundle By Name(w454) -> ("IDmap"=w451:map{string, T9}, "CmdMap"=w452:map{string, T11}, "TCP 2"=w465:refnum<k5>, "GIS Printer in"=w453:refnum<class "GIS Printer.lvclass">)
        n152 = Concatenate Strings("P,A" ("string"), "\n") -> (w464:string)
        n153 = TCP Write(connection ID=w465, data in=w464, error in (no error)=w461, 9:100 ("timeout ms (25000)")) -> (connection ID out=w458:refnum<k5>, error out=w456:errorcluster)  [unwired: 1 out]
        n154 = call-dynamic "SetPrinterBusy_Status_GIS Printer.vi"("error in (no error)"=w456, "Printer Busy?"=FALSE, "GIS Printer In"=w453) -> ("error out"=w455:errorcluster)  [unwired: 7 in, 1 out]
        n155 = for {
          tunnel: w452 -> [w476] mode=indexing
          shift-right: [w473] -> w449
          shift-left: w452 -> [w474]
          n156 = Unbundle By Name(w476) -> ("key"=w475:string)
          n157 = Remove From Map(10:w475, 11:w474) -> (3:w473:map{string, T11})  [unwired: 2 out]
        }
        n158 = for {
          tunnel: w451 -> [w472] mode=indexing
          shift-right: [w469] -> w450
          shift-left: w451 -> [w470]
          n159 = Unbundle By Name(w472) -> ("key"=w471:string)
          n160 = Remove From Map(10:w471, 11:w470) -> (3:w469:map{string, T9})  [unwired: 2 out]
        }
        n161 = call <vilib>:"Add State(s) to Queue__JKI_lib_State_Machine.vi"("State(s) in Front (\"\")"="/*Task: Remove on Error\nAction: Open Connection 2" ("State(s) in Front (\"\")")) -> ("States Out"=w467:string)  [unwired: 14 in]
        n162 = Bundle By Name(cluster=w454, "TCP 2"=w458, "IDmap"=w450, "CmdMap"=w449) -> (w459:T14)
      }
      frame "API: Execute Printer Command" {
        n163 = Unbundle By Name(w503) -> ("IDmap"=w496:map{string, T9}, "CurrentTask"=w501:T6, "TCP"=w498:refnum<k5>, "GIS Printer in"=w488:refnum<class "GIS Printer.lvclass">)
        n164 = Variant To Data(error in=w494, type=T6 {"Command"=enum."Execute Printer Command", "Arguments"=""} ("API Command Cluster"), Variant=w501) -> (data=w500:T6, error out=w495:errorcluster)
        n165 = Unbundle By Name(w500) -> ("Arguments"=w479:string)
        n166 = disable-structure shown="Enabled" {
          disable-tunnel: w498 -> [w511 w517]
          disable-tunnel: [w510 w517] -> w497
          disable-tunnel: w495 -> [w508 w514]
          disable-tunnel: w479 -> [w507 w515]
          disable-tunnel: [w506 w513] -> w486
          disable-tunnel: w477 -> [_ w512]
          frame Disabled {
            n167 = TCP Write(connection ID=w511, data in=w507, error in (no error)=w508, 9:100 ("timeout ms (25000)")) -> (connection ID out=w510:refnum<k5>, error out=w506:errorcluster)  [unwired: 1 out]
          }
          frame Enabled {
            n168 = call <vilib>:"Add State to Queue with vData.vi"("queue in"=w512, "state in"="SendCmdToPrinter", "vData (\"\")"=w515, "error in"=w514) -> ("error out"=w513:errorcluster)  [unwired: 8 in, 3 out]
          }
        }
        n169 = Get Date/Time In Seconds() -> (seconds since 1Jan1904=w482:timestamp)
        n170 = To Double Precision Float(number=w482) -> (double precision float=w491:dbl)
        n171 = Bundle By Name(cluster=T9 {"WaitFor"="", "SentTime"=0.0, "PrinterCmdStatus"=enum."WaitingForAck"} ("value"), "WaitFor"=w479, "SentTime"=w491, "PrinterCmdStatus"=PrinterCmdStatus--Enum."WaitingForAck") -> (w490:T9)
        n172 = Format Date/Time String(seconds (now)=w482) -> (date/time string=w481:string)  [unwired: 2 in]
        n173 = call-dynamic "SetCommandStatus_GIS Printer.vi"("error in (no error)"=w486, "Command Data"=T3 {"PrinterResponse"="", "Cmd Status"=enum."WaitingForAck"}, "Command"=w479, "GIS Printer In"=w488) -> ("error out"=w484:errorcluster, "GIS Printer Out"=w485:refnum<class "GIS Printer.lvclass">)  [unwired: 6 in]
        n174 = Insert Into Map(map in=w496, key=w479, value=w490) -> (map out=w493:map{string, T9})  [unwired: 2 out]
        n175 = Build Array(w481, "-->", w479) -> (w478:string[])
        n176 = Bundle By Name(cluster=w503, "IDmap"=w493, "TCP"=w497) -> (w499:T14)
        n177 = call-dynamic "AddTCPCommands&Responses_GIS Printer.vi"("error in (no error)"=w484, "Command \\ Response"=w478, "GIS Printer In"=w485) -> ("error out"=w483:errorcluster)  [unwired: 7 in, 1 out]
      }
      frame "---------- Action ----------" {
      }
      frame "Action: Launch Abort Process" {
        n178 = Unbundle By Name(w524) -> ("GIS Printer in"=w523:refnum<class "GIS Printer.lvclass">)
        n179 = vi-ref "GIS Printer.lvclass:AbortProcess.vi"() -> (w533:refnum<vi>)
        n180 = property class="VI"(reference=w533) -> ("Name"=w532:string)  [unwired: 1 in, 2 out]
        n181 = Open VI Reference(type specifier VI Refnum (for type only)=refnum<vi> refnum, vi path=w532, options=128, error in (no error)=w525) -> (vi reference=w529:refnum<vi>, error out=w528:errorcluster)  [unwired: 2 in]
        n182 = call-by-ref "Start Asynchronous Call"(reference=w529, error in=w528, 8:"error in (no error)"=w528, "TopLevel"=w522, "GIS Printer in"=w523) -> (reference out=w527:refnum<vi>, error out=w526:errorcluster)  [unwired: 7 in, 2 out]
        n183 = Close Reference(reference=w527, error in (no error)=w526) -> ()  [unwired: 1 out]
      }
      frame "Move Stage" {
        n184 = Unbundle By Name(w541) -> ("PrinterConfiguration.Move Stage on RTP Command?"=w540:bool, "Motor Controller"=w538:refnum<class "Motor Controller.lvclass">)
        n185 = case shown="True" w540 {
          tunnel: w539 -> [w544 w548]
          tunnel: w536 -> [_ w546]
          tunnel: w538 -> [_ w545]
          tunnel: [w544 w547] -> w537
          frame False {
          }
          frame True {
            n186 = case shown="\"Laminate\"" w546 {
              tunnel: w548 -> [w549 w550 w555]
              tunnel: [w549 w551 w556] -> w547
              tunnel: w545 -> [_ w552 w557]
              frame Default {
              }
              frame "Laminate" {
                n187 = call "Laminate API.vi"("error in (no error)"=w550, "Motor Controller in"=w552) -> ("error out"=w551:errorcluster)  [unwired: 7 in, 2 out]
              }
              frame "Home" {
                n188 = call "API_HomeStage.vi"("Timeout (ms)"=u32 600000, "Wait (F)"=TRUE, "error in (no error)"=w555, "Motor Controller in"=w557) -> ("error out"=w556:errorcluster)  [unwired: 5 in, 2 out]
              }
            }
          }
        }
      }
      frame "---------- Tasks ----------" {
      }
      frame "Action: Open Connection" {
        n189 = disable-structure shown="Enabled" {
          disable-tunnel: w568 -> [w578 w579]
          disable-tunnel: w567 -> [w577 _]
          disable-tunnel: [w575 w579] -> w566
          disable-tunnel: [w574 refnum<k5> refnum ("connection ID")] -> w563
          frame Enabled {
            (unwired) "localhost" ("address")
            n190 = Unbundle By Name(w577) -> ("PrinterConfiguration.IPAddress"=w572:string)
            n191 = TCP Open Connection(address=w572, remote port or service name=u16 2000, timeout ms (60000)=1000, error in (no error)=w578) -> (connection ID=w574:refnum<k5>, error out=w575:errorcluster)  [unwired: 1 in]
          }
          frame Disabled {
          }
        }
        n192 = call <vilib>:"Add State to Queue with vData.vi"("queue in"=w564, "state in"="UpdateSettings>>TCP", "vData (\"\")"=w563, "error in"=w566) -> ("error out"=w565:errorcluster)  [unwired: 8 in, 3 out]
        n193 = Bundle By Name(cluster=w567, "TCP"=w563) -> (w569:T14)
      }
      frame "Action: Open Connection 2" {
        n194 = disable-structure shown="Enabled" {
          disable-tunnel: w587 -> [w597 w598]
          disable-tunnel: w586 -> [w596 _]
          disable-tunnel: [w594 w598] -> w585
          disable-tunnel: [w593 refnum<k5> refnum ("connection ID")] -> w582
          frame Enabled {
            (unwired) "localhost" ("address")
            n195 = Unbundle By Name(w596) -> ("PrinterConfiguration.IPAddress"=w591:string)
            n196 = TCP Open Connection(address=w591, remote port or service name=u16 2000, timeout ms (60000)=1000, error in (no error)=w597) -> (connection ID=w593:refnum<k5>, error out=w594:errorcluster)  [unwired: 1 in]
          }
          frame Disabled {
          }
        }
        n197 = call <vilib>:"Add State to Queue with vData.vi"("queue in"=w583, "state in"="UpdateSettings>>TCP 2", "vData (\"\")"=w582, "error in"=w585) -> ("error out"=w584:errorcluster)  [unwired: 8 in, 3 out]
        n198 = Bundle By Name(cluster=w586, "TCP 2"=w582) -> (w588:T14)
      }
      frame "Action: Close Connection" {
        n199 = Unbundle By Name(w605) -> ("TCP"=w602:refnum<k5>, "TCP 2"=w601:refnum<k5>)
        n200 = disable-structure shown="Enabled" {
          disable-tunnel: w604 -> [w610 w613]
          disable-tunnel: [w612 w613] -> w603
          disable-tunnel: w602 -> [w611 _]
          disable-tunnel: w601 -> [w609 _]
          frame Enabled {
            n201 = TCP Close Connection(connection ID=w611, error in (no error)=w610) -> (error out=w612:errorcluster)  [unwired: 1 in, 1 out]
            n202 = TCP Close Connection(connection ID=w609, error in (no error)=w610) -> (error out=w608:errorcluster)  [unwired: 1 in, 1 out]
            n203 = call <userlib>:"MGI Clear Error.vi"("Error In"=w608) -> ()  [unwired: 6 in, 1 out]
          }
          frame Disabled {
          }
        }
        n204 = call <vilib>:"Clear Errors.vi"("error in (no error)"=w603) -> ("error out"=w600:errorcluster)  [unwired: 5 in, 1 out]
      }
      frame "Task: Completed" {
        n205 = Unbundle By Name(w620) -> ("API Executed Event"=w618:refnum<user-event>, "Tasks"=w617:T4[], "Current Task. Return Value"=w614:variant)
        n206 = Empty Array?(array=w617) -> (empty?=w619:bool)
        n207 = case shown="False" w619 {
          tunnel: w618 -> [w629 _]
          tunnel: w617 -> [w630 _]
          tunnel: w615 -> [w627 w631]
          tunnel: [w626 w631] -> w616
          tunnel: w614 -> [w624 _]
          frame False {
            n208 = Index Array(array=w630) -> (element=w628:T4)  [unwired: 1 in]
            n209 = Bundle By Name(cluster=w628, "Task.Task State"=API_Task_State."Completed", "Return Value"=w624) -> (w625:T4)
            n210 = Generate User Event(user event=w629, event data cluster=w625, error in=w627) -> (error out=w626:errorcluster)  [unwired: 1 in, 1 out]
          }
          frame True {
          }
        }
      }
      frame "Task: Check Timeout" {
        n211 = Unbundle By Name(w640) -> ("API Executed Event"=w638:refnum<user-event>, "Task Start ms"=w633:u32, "Tasks"=w635:T4[])
        n212 = Index Array(array=w635) -> (element=w634:T4)  [unwired: 1 in]
        n213 = Empty Array?(array=w635) -> (empty?=w639:bool)
        n214 = case shown="True" w639 {
          tunnel: w638 -> [w644 _]
          tunnel: w636 -> [w650 w659]
          tunnel: [w645 w660] -> w637
          tunnel: w634 -> [w649 _]
          tunnel: w633 -> [w653 _]
          tunnel: w632 -> [_ w661]
          frame False {
            n215 = Unbundle By Name(w649) -> ("Task.Timeout (ms)"=w651:u32)
            n216 = Tick Count (ms)() -> (millisecond timer value=w643:u32)
            n217 = Subtract(x=w643, y=w653) -> (x-y=w652:u32)
            n218 = Bundle By Name(cluster=w649, "Task.Task State"=API_Task_State."Errored") -> (w647:T4)
            n219 = Greater Or Equal?(x=w652, y=w651) -> (x >= y?=w646:bool)
            n220 = case shown="True" w646 {
              tunnel: w650 -> [w654 w658]
              tunnel: w647 -> [_ w656]
              tunnel: [w654 w657] -> w645
              tunnel: w644 -> [_ w655]
              frame False {
              }
              frame True {
                n221 = Generate User Event(user event=w655, event data cluster=w656, error in=w658) -> (error out=w657:errorcluster)  [unwired: 1 in, 1 out]
              }
            }
          }
          frame True {
            n222 = call-dynamic "SetPrinterBusy_Status_GIS Printer.vi"("error in (no error)"=w659, "Printer Busy?"=FALSE, "GIS Printer In"=w661) -> ("error out"=w660:errorcluster)  [unwired: 7 in, 1 out]
          }
        }
      }
      frame "Task: Check Pending" {
        n223 = Unbundle By Name(w664) -> ("API Executed Event"=w673:refnum<user-event>, "Task Start ms"=w670:u32, "Tasks"=w669:T4[])
        n224 = Empty Array?(array=w669) -> (empty?=w674:bool)
        n225 = case shown="False" w674 {
          tunnel: w673 -> [_ _]
          tunnel: w671 -> [w684 w692]
          tunnel: [w682 w693] -> w672
          tunnel: w670 -> [_ _]
          tunnel: w669 -> [w691 _]
          tunnel: [w681 _] -> w666
          tunnel: w664 -> [w680 w696]
          tunnel: [w678 w696] -> w665
          tunnel: w663 -> [_ w694]
          frame False {
            n226 = Index Array(array=w691) -> (element=w686:T4)  [unwired: 1 in]
            n227 = Unbundle By Name(w686) -> ("Command"=w685:variant)
            n228 = Variant To Data(error in=w684, type=T6 {"Command"=enum."Execute Printer Command", "Arguments"=""} ("API Command Cluster"), Variant=w685) -> (data=w676:T6, error out=w683:errorcluster)
            n229 = Unbundle By Name(w676) -> ("Command"=w688:T7, "Arguments"=w687:string)
            n230 = Tick Count (ms)() -> (millisecond timer value=w679:u32)
            n231 = Bundle By Name(cluster=w680, "TO"=100, "Task Start ms"=w679, "CurrentTask"=w676) -> (w678:T14)
            n232 = Format Into String(format string="API: %s>>%s", error in=w683, w688, w687) -> (resulting string=w681:string, error out=w682:errorcluster)  [unwired: 1 in]
          }
          frame True {
            n233 = call-dynamic "SetPrinterBusy_Status_GIS Printer.vi"("error in (no error)"=w692, "Printer Busy?"=FALSE, "GIS Printer In"=w694) -> ("error out"=w693:errorcluster)  [unwired: 7 in, 1 out]
          }
        }
        n234 = call <vilib>:"Add State(s) to Queue__JKI_lib_State_Machine.vi"("State(s) in Front (\"\")"=w666, "State(s) in (\"\")"=w667) -> ("States Out"=w668:string)  [unwired: 13 in]
      }
      frame "Task: Remove on Error" {
        n235 = Unbundle By Name(w702) -> ("API Return Event"=w704:refnum<user-event>, "Tasks"=w703:T4[])
        n236 = for {
          tunnel: w704 -> [w714]
          tunnel: w703 -> [w713] mode=indexing
          shift-right: [w708] -> w701
          shift-left: w700 -> [w709]
          n237 = Get Date/Time In Seconds() -> (seconds since 1Jan1904=w710:timestamp)
          n238 = Bundle By Name(cluster=w713, "Task.Task State"=API_Task_State."Errored", "Task.Time Stamp"=w710) -> (w712:T4)
          n239 = Generate User Event(user event=w714, event data cluster=w712, error in=w709) -> (error out=w708:errorcluster)  [unwired: 1 in, 1 out]
        }
        n240 = Bundle By Name(cluster=w702, "TO"=100, "Tasks"=T4[] []) -> (w699:T14)
        n241 = call <vilib>:"Add State(s) to Queue__JKI_lib_State_Machine.vi"("State(s) in (\"\")"=w705) -> ("States Out"=w706:string)  [unwired: 14 in]
      }
    }
  }
  "error out" <- w12
  n242 = Bundle By Name(cluster=T1 {"String"="", "PrinterResponse"=refnum, "TCP"=refnum, "Open"=FALSE, "TCP 2"=refnum, "Open 2"=FALSE}, "PrinterResponse"=w3) -> (w4:T1)
  n243 = disable-structure shown="Enabled" {
    disable-tunnel: w8 -> [w717 w851 w1157]
    disable-tunnel: w4 -> [w716 w850 w1156]
    disable-tunnel: w2 -> [w715 w849 w1155]
    frame Enabled {
      n244 = while {
        tunnel: w715 -> [w723]
        shift-right: [w727] -> _
        shift-left: w717 -> [w729]
        shift-right: [w724] -> _
        shift-left: w716 -> [w725]
        stop <- w730 stop-if-true
        n245 = call <vilib>:"Get Next Queued State with vData.vi"("queue in"=w723, "error in (no error)"=w729) -> ("vData out"=w726:variant, "queue out"=w722:refnum<queue>, "Next State"=w721:string, "queued msg"=w718:string, "error out"=w728:errorcluster)  [unwired: 7 in, 2 out]
        n246 = call <vilib>:"Parse State Queue__JKI_lib_State_Machine.vi"("State Queue"=w721) -> ("Current State"=w720:string, "Arguments"=w719:string)  [unwired: 12 in, 1 out]
        n247 = case shown="\"\", \"EventHandler\", \"Idle\"" w720 {
          tunnel: [_ _ _ _ _ _ _ TRUE] -> w730
          tunnel: w728 -> [w732 w745 w769 w773 w808 w814 w842 w847]
          tunnel: [w732 w735 w769 w772 errorcluster {"status"=FALSE, "code"=0, "source"=""} ("error out") w813 w841 w847] -> w727
          tunnel: w726 -> [_ w743 _ _ _ w815 _ _]
          tunnel: w725 -> [w731 w740 w768 w771 w807 w812 w845 w846]
          tunnel: [w731 w738 w767 w770 w807 w811 w840 w846] -> w724
          tunnel: w722 -> [_ _ _ _ _ _ w844 _]
          tunnel: w719 -> [_ _ _ _ _ _ _ _]
          tunnel: w718 -> [_ _ _ _ _ w810 _ _]
          frame Default {
          }
          frame "SendCmdToPrinter" {
            n248 = Variant To Data(error in=w745, type="", Variant=w743) -> (data=w742:string, error out=w741:errorcluster)
            n249 = Unbundle By Name(w740) -> ("TCP"=w739:refnum<k5>)
            n250 = Concatenate Strings(w742, "\n") -> (w734:string)
            n251 = disable-structure shown="Enabled" {
              disable-tunnel: w739 -> [w763 w765]
              disable-tunnel: [w762 w765] -> w737
              disable-tunnel: w741 -> [w760 w764]
              disable-tunnel: w734 -> [w759 _]
              disable-tunnel: [w758 w764] -> w736
              disable-tunnel: [w757 _] -> _
              frame Enabled {
                n252 = TCP Write(connection ID=w763, data in=w759, error in (no error)=w760, 9:100 ("timeout ms (25000)")) -> (connection ID out=w762:refnum<k5>, bytes written=w757:i32, error out=w758:errorcluster)
              }
              frame Disabled {
              }
            }
            n253 = disable-structure shown="Enabled" {
              disable-tunnel: w740 -> [w754 w756]
              disable-tunnel: [w753 w756] -> w738
              disable-tunnel: w737 -> [w750 _]
              disable-tunnel: w736 -> [w749 w755]
              disable-tunnel: [w748 w755] -> w735
              frame Disabled {
                n254 = TCP Read(connection ID=w750, bytes to read=100, error in (no error)=w749, 9:1000 ("timeout ms (25000)")) -> (connection ID out=w746:refnum<k5>, data out=w747:string, error out=w748:errorcluster)  [unwired: 1 in]
                n255 = Bundle By Name(cluster=w754, "TCP"=w746) -> (w753:T1)
                n256 = flat-sequence {
                  tunnel: w747 -> [_]
                  frame #0 {
                  }
                }
              }
              frame Enabled {
              }
            }
          }
          frame "Initialize" {
            n257 = Bundle By Name(cluster=w768, "Open"=FALSE) -> (w767:T1)
          }
          frame "", "EventHandler", "Idle" {
            n258 = event shown="[0] Timeout" {
              selector: _ -> [_]
              dyn-events: _ -> [_]
              timeout: 1 -> [_]
              tunnel: w771 -> [w778]
              tunnel: w773 -> [w776]
              tunnel: [w775] -> w772
              tunnel: [w779] -> w770
              event Timeout {
                n259 = event-data() -> ()  [unwired: 1 in, 3 out]
                n260 = Unbundle By Name(w778) -> ("Open"=w777:bool)
                n261 = case shown="True" w777 {
                  tunnel: w778 -> [w781 w795]
                  tunnel: [w781 w793] -> w779
                  tunnel: w776 -> [w780 w783]
                  tunnel: [w780 w782] -> w775
                  frame False {
                  }
                  frame True {
                    n262 = Unbundle By Name(w795) -> ("String"=w794:string, "PrinterResponse"=w791:refnum<user-event>, "TCP"=w790:refnum<k5>)
                    n263 = TCP Read(connection ID=w790, bytes to read=500, error in (no error)=w783, 9:100 ("timeout ms (25000)")) -> (connection ID out=w784:refnum<k5>, data out=w789:string, error out=w785:errorcluster)  [unwired: 1 in]
                    n264 = Empty String/Path?(string/path=w789) -> (empty?=w788:bool)
                    n265 = case shown="True" w788 {
                      tunnel: w794 -> [w802 w805]
                      tunnel: [w801 w806] -> w792
                      tunnel: w791 -> [w800 w804]
                      tunnel: w789 -> [w799 _]
                      frame False {
                        n266 = Concatenate Strings(w802, w799) -> (w803:string)
                        n267 = call "ProcessSerialData.vi"("SerialResponseEvent"=w800, "String in"=w803) -> ("String out"=w801:string)  [unwired: 9 in]
                      }
                      frame True {
                        n268 = call "ProcessSerialData.vi"("SerialResponseEvent"=w804, "String in"=w805) -> ("String out"=w806:string)  [unwired: 9 in]
                      }
                    }
                    n269 = flat-sequence {
                      tunnel: w785 -> [w798]
                      tunnel: [w796] -> w782
                      frame #0 {
                        # "#todo handle error 56"
                        n270 = call <vilib>:"Clear Errors.vi"("error in (no error)"=w798, "specific error code to clear (0: all)"=56) -> ("error out"=w796:errorcluster)  [unwired: 4 in, 1 out]
                      }
                    }
                    n271 = Bundle By Name(cluster=w795, "String"=w792, "TCP"=w784) -> (w793:T1)
                  }
                }
              }
            }
          }
          frame "Error Handler" {
            n272 = call <vilib>:"General Error Handler.vi"("error in (no error)"=w808) -> ()  [unwired: 10 in, 5 out]
          }
          frame "UpdateSettings" {
            n273 = case shown="\"TCP\"" w810 {
              tunnel: w815 -> [_ w819 w827 w835]
              tunnel: w814 -> [w817 w820 w828 w836]
              tunnel: [w817 w821 w829 w837] -> w813
              tunnel: w812 -> [w816 w822 w830 w838]
              tunnel: [w816 w822 w825 w833] -> w811
              frame "False", Default {
              }
              frame "Configuration" {
                n274 = Variant To Data(error in=w820, type="placeholder", Variant=w819) -> (error out=w821:errorcluster)  [unwired: 1 out]
              }
              frame "TCP" {
                w826 = refnum<k5> refnum  # TCP
                n275 = Variant To Data(error in=w828, type=w826, Variant=w827) -> (data=w824:refnum<k5>, error out=w829:errorcluster)
                n276 = Bundle By Name(cluster=w830, "TCP"=w824, "Open"=TRUE) -> (w825:T1)
              }
              frame "TCP 2" {
                w834 = refnum<k5> refnum  # TCP
                n277 = Variant To Data(error in=w836, type=w834, Variant=w835) -> (data=w832:refnum<k5>, error out=w837:errorcluster)
                n278 = Bundle By Name(cluster=w838, "TCP 2"=w832, "Open 2"=TRUE ("Open")) -> (w833:T1)
              }
            }
          }
          frame "Macro: Exit" {
            w839 = FALSE ("Open")
            n279 = Bundle By Name(cluster=w845, "Open"=w839, "Open 2"=w839) -> (w840:T1)
            n280 = call <vilib>:"Add States to Queue using MultiLine String (no vData input).vi"("queue in"=w844, "states in"="Quit", "error in"=w842) -> ("error out"=w841:errorcluster)  [unwired: 10 in, 2 out]
          }
          frame "Quit" {
          }
        }
      }
    }
    frame Disabled {
      n281 = while {
        tunnel: w849 -> [w857]
        shift-right: [w861] -> _
        shift-left: w851 -> [w863]
        shift-right: [w858] -> _
        shift-left: w850 -> [w859]
        stop <- w864 stop-if-true
        n282 = call <vilib>:"Get Next Queued State with vData.vi"("queue in"=w857, "error in (no error)"=w863) -> ("vData out"=w860:variant, "queue out"=w856:refnum<queue>, "Next State"=w855:string, "queued msg"=w852:string, "error out"=w862:errorcluster)  [unwired: 7 in, 2 out]
        n283 = call <vilib>:"Parse State Queue__JKI_lib_State_Machine.vi"("State Queue"=w855) -> ("Current State"=w854:string, "Arguments"=w853:string)  [unwired: 12 in, 1 out]
        n284 = case shown="\"\", \"EventHandler\", \"Idle\"" w854 {
          tunnel: [_ _ _ _ _ _ _ TRUE] -> w864
          tunnel: w862 -> [w866 w879 w903 w907 w1124 w1130 w1148 w1153]
          tunnel: [w866 w869 w903 w906 errorcluster {"status"=FALSE, "code"=0, "source"=""} ("error out") w1129 w1147 w1153] -> w861
          tunnel: w860 -> [_ w877 _ _ _ w1131 _ _]
          tunnel: w859 -> [w865 w874 w902 w905 w1123 w1128 w1151 w1152]
          tunnel: [w865 w872 w901 w904 w1123 w1127 w1151 w1152] -> w858
          tunnel: w856 -> [_ _ _ _ _ _ w1150 _]
          tunnel: w853 -> [_ _ _ _ _ _ _ _]
          tunnel: w852 -> [_ _ _ _ _ w1126 _ _]
          frame Default {
          }
          frame "SendCmdToPrinter" {
            n285 = Variant To Data(error in=w879, type="", Variant=w877) -> (data=w876:string, error out=w875:errorcluster)
            n286 = Unbundle By Name(w874) -> ("TCP"=w873:refnum<k5>)
            n287 = Concatenate Strings(w876, "\n") -> (w868:string)
            n288 = disable-structure shown="Enabled" {
              disable-tunnel: w873 -> [w897 w899]
              disable-tunnel: [w896 w899] -> w871
              disable-tunnel: w875 -> [w894 w898]
              disable-tunnel: w868 -> [w893 _]
              disable-tunnel: [w892 w898] -> w870
              disable-tunnel: [w891 _] -> _
              frame Disabled {
                n289 = TCP Write(connection ID=w897, data in=w893, error in (no error)=w894, 9:100 ("timeout ms (25000)")) -> (connection ID out=w896:refnum<k5>, bytes written=w891:i32, error out=w892:errorcluster)
              }
              frame Enabled {
              }
            }
            n290 = disable-structure shown="Enabled" {
              disable-tunnel: w874 -> [w888 w890]
              disable-tunnel: [w887 w890] -> w872
              disable-tunnel: w871 -> [w884 _]
              disable-tunnel: w870 -> [w883 w889]
              disable-tunnel: [w882 w889] -> w869
              frame Disabled {
                n291 = TCP Read(connection ID=w884, bytes to read=100, error in (no error)=w883, 9:1000 ("timeout ms (25000)")) -> (connection ID out=w880:refnum<k5>, data out=w881:string, error out=w882:errorcluster)  [unwired: 1 in]
                n292 = Bundle By Name(cluster=w888, "TCP"=w880) -> (w887:T1)
                n293 = flat-sequence {
                  tunnel: w881 -> [_]
                  frame #0 {
                  }
                }
              }
              frame Enabled {
              }
            }
          }
          frame "Initialize" {
            n294 = Bundle By Name(cluster=w902, "Open"=FALSE) -> (w901:T1)
          }
          frame "", "EventHandler", "Idle" {
            n295 = event shown="[0] Timeout" {
              selector: _ -> [_ _ _ _ _ _ _ _ _ _]
              dyn-events: _ -> [_ _ _ _ _ _ _ _ _ _]
              timeout: 1 -> [_ _ _ _ _ _ _ _ _ _]
              tunnel: w905 -> [w910 w935 w956 w977 w998 w1019 w1040 w1061 w1082 w1103]
              tunnel: w907 -> [w912 w937 w958 w979 w1000 w1021 w1042 w1063 w1084 w1105]
              tunnel: [w912 w937 w958 w979 w1000 w1021 w1042 w1063 w1084 w1105] -> w906
              tunnel: [w911 w936 w957 w978 w999 w1020 w1041 w1062 w1083 w1104] -> w904
              event Timeout {
                n296 = event-data() -> ()  [unwired: 1 in, 3 out]
                n297 = Unbundle By Name(w910) -> ("Open"=w909:bool)
                n298 = case shown="True" w909 {
                  tunnel: w910 -> [w913 w925]
                  tunnel: [w913 w923] -> w911
                  frame False {
                  }
                  frame True {
                    n299 = Unbundle By Name(w925) -> ("String"=w924:string, "PrinterResponse"=w921:refnum<user-event>, "TCP"=w920:refnum<k5>)
                    n300 = TCP Read(connection ID=w920, bytes to read=500, 9:100 ("timeout ms (25000)")) -> (connection ID out=w914:refnum<k5>, data out=w919:string, error out=w915:errorcluster)  [unwired: 2 in]
                    n301 = Empty String/Path?(string/path=w919) -> (empty?=w918:bool)
                    n302 = case shown="False" w918 {
                      tunnel: w924 -> [w929 w932]
                      tunnel: [w928 w933] -> w922
                      tunnel: w921 -> [w927 w931]
                      tunnel: w919 -> [w926 _]
                      frame False {
                        n303 = Concatenate Strings(w929, w926) -> (w930:string)
                        n304 = call "ProcessSerialData.vi"("SerialResponseEvent"=w927, "String in"=w930) -> ("String out"=w928:string)  [unwired: 9 in]
                      }
                      frame True {
                        n305 = call "ProcessSerialData.vi"("SerialResponseEvent"=w931, "String in"=w932) -> ("String out"=w933:string)  [unwired: 9 in]
                      }
                    }
                    n306 = flat-sequence {
                      tunnel: w915 -> [_]
                      frame #0 {
                        # "#todo handle error 56"
                      }
                    }
                    n307 = Bundle By Name(cluster=w925, "String"=w922, "TCP"=w914) -> (w923:T1)
                  }
                }
              }
              event "A11": Value Change {
                n308 = event-data() -> ()  [unwired: 1 in, 6 out]
                n309 = Unbundle By Name(w935) -> ("Open"=w934:bool)
                n310 = case shown="True" w934 {
                  tunnel: w935 -> [w938 w946]
                  tunnel: [w938 w944] -> w936
                  frame False {
                  }
                  frame True {
                    w939 = "A,11,P,C,P,\"Print Manager,Print Line Manager,PMB-KM,PrintGoSource\",\"TTL\"\n"
                    n311 = Unbundle By Name(w946) -> ("String"=w945:string, "PrinterResponse"=w942:refnum<user-event>, "TCP"=w940:refnum<k5>)
                    n312 = Empty String/Path?(string/path=w939) -> (empty?=w941:bool)
                    n313 = case shown="False" w941 {
                      tunnel: w945 -> [w950 w953]
                      tunnel: [w949 w954] -> w943
                      tunnel: w942 -> [w948 w952]
                      tunnel: w939 -> [w947 _]
                      frame False {
                        n314 = Concatenate Strings(w950, w947) -> (w951:string)
                        n315 = call "ProcessSerialData.vi"("SerialResponseEvent"=w948, "String in"=w951) -> ("String out"=w949:string)  [unwired: 9 in]
                      }
                      frame True {
                        n316 = call "ProcessSerialData.vi"("SerialResponseEvent"=w952, "String in"=w953) -> ("String out"=w954:string)  [unwired: 9 in]
                      }
                    }
                    n317 = Bundle By Name(cluster=w946, "String"=w943, "TCP"=w940) -> (w944:T1)
                  }
                }
              }
              event "C11": Value Change {
                n318 = event-data() -> ()  [unwired: 1 in, 6 out]
                n319 = Unbundle By Name(w956) -> ("Open"=w955:bool)
                n320 = case shown="True" w955 {
                  tunnel: w956 -> [w959 w967]
                  tunnel: [w959 w965] -> w957
                  frame False {
                  }
                  frame True {
                    w960 = "C,11,0\n"
                    n321 = Unbundle By Name(w967) -> ("String"=w966:string, "PrinterResponse"=w963:refnum<user-event>, "TCP"=w961:refnum<k5>)
                    n322 = Empty String/Path?(string/path=w960) -> (empty?=w962:bool)
                    n323 = case shown="True" w962 {
                      tunnel: w966 -> [w971 w974]
                      tunnel: [w970 w975] -> w964
                      tunnel: w963 -> [w969 w973]
                      tunnel: w960 -> [w968 _]
                      frame False {
                        n324 = Concatenate Strings(w971, w968) -> (w972:string)
                        n325 = call "ProcessSerialData.vi"("SerialResponseEvent"=w969, "String in"=w972) -> ("String out"=w970:string)  [unwired: 9 in]
                      }
                      frame True {
                        n326 = call "ProcessSerialData.vi"("SerialResponseEvent"=w973, "String in"=w974) -> ("String out"=w975:string)  [unwired: 9 in]
                      }
                    }
                    n327 = Bundle By Name(cluster=w967, "String"=w964, "TCP"=w961) -> (w965:T1)
                  }
                }
              }
              event "A22": Value Change {
                n328 = event-data() -> ()  [unwired: 1 in, 6 out]
                n329 = Unbundle By Name(w977) -> ("Open"=w976:bool)
                n330 = case shown="True" w976 {
                  tunnel: w977 -> [w980 w988]
                  tunnel: [w980 w986] -> w978
                  frame False {
                  }
                  frame True {
                    w981 = "A,22,P,C,P,\"Print Manager,Print Line Manager,PMB-KM,EncoderSource\",\"RS422\"\n"
                    n331 = Unbundle By Name(w988) -> ("String"=w987:string, "PrinterResponse"=w984:refnum<user-event>, "TCP"=w982:refnum<k5>)
                    n332 = Empty String/Path?(string/path=w981) -> (empty?=w983:bool)
                    n333 = case shown="True" w983 {
                      tunnel: w987 -> [w992 w995]
                      tunnel: [w991 w996] -> w985
                      tunnel: w984 -> [w990 w994]
                      tunnel: w981 -> [w989 _]
                      frame False {
                        n334 = Concatenate Strings(w992, w989) -> (w993:string)
                        n335 = call "ProcessSerialData.vi"("SerialResponseEvent"=w990, "String in"=w993) -> ("String out"=w991:string)  [unwired: 9 in]
                      }
                      frame True {
                        n336 = call "ProcessSerialData.vi"("SerialResponseEvent"=w994, "String in"=w995) -> ("String out"=w996:string)  [unwired: 9 in]
                      }
                    }
                    n337 = Bundle By Name(cluster=w988, "String"=w985, "TCP"=w982) -> (w986:T1)
                  }
                }
              }
              event "C22": Value Change {
                n338 = event-data() -> ()  [unwired: 1 in, 6 out]
                n339 = Unbundle By Name(w998) -> ("Open"=w997:bool)
                n340 = case shown="True" w997 {
                  tunnel: w998 -> [w1001 w1009]
                  tunnel: [w1001 w1007] -> w999
                  frame False {
                  }
                  frame True {
                    w1002 = "C,22,0\n"
                    n341 = Unbundle By Name(w1009) -> ("String"=w1008:string, "PrinterResponse"=w1005:refnum<user-event>, "TCP"=w1003:refnum<k5>)
                    n342 = Empty String/Path?(string/path=w1002) -> (empty?=w1004:bool)
                    n343 = case shown="True" w1004 {
                      tunnel: w1008 -> [w1013 w1016]
                      tunnel: [w1012 w1017] -> w1006
                      tunnel: w1005 -> [w1011 w1015]
                      tunnel: w1002 -> [w1010 _]
                      frame False {
                        n344 = Concatenate Strings(w1013, w1010) -> (w1014:string)
                        n345 = call "ProcessSerialData.vi"("SerialResponseEvent"=w1011, "String in"=w1014) -> ("String out"=w1012:string)  [unwired: 9 in]
                      }
                      frame True {
                        n346 = call "ProcessSerialData.vi"("SerialResponseEvent"=w1015, "String in"=w1016) -> ("String out"=w1017:string)  [unwired: 9 in]
                      }
                    }
                    n347 = Bundle By Name(cluster=w1009, "String"=w1006, "TCP"=w1003) -> (w1007:T1)
                  }
                }
              }
              event "A33": Value Change {
                n348 = event-data() -> ()  [unwired: 1 in, 6 out]
                n349 = Unbundle By Name(w1019) -> ("Open"=w1018:bool)
                n350 = case shown="True" w1018 {
                  tunnel: w1019 -> [w1022 w1030]
                  tunnel: [w1022 w1028] -> w1020
                  frame False {
                  }
                  frame True {
                    w1023 = "A,33,P,P,1,C:\\Users\\labuser\\Desktop\\Scripts\\Patterns\\Print Weights\\PH1\\PW.bmp,5\n"
                    n351 = Unbundle By Name(w1030) -> ("String"=w1029:string, "PrinterResponse"=w1026:refnum<user-event>, "TCP"=w1024:refnum<k5>)
                    n352 = Empty String/Path?(string/path=w1023) -> (empty?=w1025:bool)
                    n353 = case shown="True" w1025 {
                      tunnel: w1029 -> [w1034 w1037]
                      tunnel: [w1033 w1038] -> w1027
                      tunnel: w1026 -> [w1032 w1036]
                      tunnel: w1023 -> [w1031 _]
                      frame False {
                        n354 = Concatenate Strings(w1034, w1031) -> (w1035:string)
                        n355 = call "ProcessSerialData.vi"("SerialResponseEvent"=w1032, "String in"=w1035) -> ("String out"=w1033:string)  [unwired: 9 in]
                      }
                      frame True {
                        n356 = call "ProcessSerialData.vi"("SerialResponseEvent"=w1036, "String in"=w1037) -> ("String out"=w1038:string)  [unwired: 9 in]
                      }
                    }
                    n357 = Bundle By Name(cluster=w1030, "String"=w1027, "TCP"=w1024) -> (w1028:T1)
                  }
                }
              }
              event "I33 1": Value Change {
                n358 = event-data() -> ()  [unwired: 1 in, 6 out]
                n359 = Unbundle By Name(w1040) -> ("Open"=w1039:bool)
                n360 = case shown="True" w1039 {
                  tunnel: w1040 -> [w1043 w1051]
                  tunnel: [w1043 w1049] -> w1041
                  frame False {
                  }
                  frame True {
                    w1044 = "I,33,P\n"
                    n361 = Unbundle By Name(w1051) -> ("String"=w1050:string, "PrinterResponse"=w1047:refnum<user-event>, "TCP"=w1045:refnum<k5>)
                    n362 = Empty String/Path?(string/path=w1044) -> (empty?=w1046:bool)
                    n363 = case shown="True" w1046 {
                      tunnel: w1050 -> [w1055 w1058]
                      tunnel: [w1054 w1059] -> w1048
                      tunnel: w1047 -> [w1053 w1057]
                      tunnel: w1044 -> [w1052 _]
                      frame False {
                        n364 = Concatenate Strings(w1055, w1052) -> (w1056:string)
                        n365 = call "ProcessSerialData.vi"("SerialResponseEvent"=w1053, "String in"=w1056) -> ("String out"=w1054:string)  [unwired: 9 in]
                      }
                      frame True {
                        n366 = call "ProcessSerialData.vi"("SerialResponseEvent"=w1057, "String in"=w1058) -> ("String out"=w1059:string)  [unwired: 9 in]
                      }
                    }
                    n367 = Bundle By Name(cluster=w1051, "String"=w1048, "TCP"=w1045) -> (w1049:T1)
                  }
                }
              }
              event "I33 2": Value Change {
                n368 = event-data() -> ()  [unwired: 1 in, 6 out]
                n369 = Unbundle By Name(w1061) -> ("Open"=w1060:bool)
                n370 = case shown="True" w1060 {
                  tunnel: w1061 -> [w1064 w1072]
                  tunnel: [w1064 w1070] -> w1062
                  frame False {
                  }
                  frame True {
                    w1065 = "I,33,RTP,1\n"
                    n371 = Unbundle By Name(w1072) -> ("String"=w1071:string, "PrinterResponse"=w1068:refnum<user-event>, "TCP"=w1066:refnum<k5>)
                    n372 = Empty String/Path?(string/path=w1065) -> (empty?=w1067:bool)
                    n373 = case shown="True" w1067 {
                      tunnel: w1071 -> [w1076 w1079]
                      tunnel: [w1075 w1080] -> w1069
                      tunnel: w1068 -> [w1074 w1078]
                      tunnel: w1065 -> [w1073 _]
                      frame False {
                        n374 = Concatenate Strings(w1076, w1073) -> (w1077:string)
                        n375 = call "ProcessSerialData.vi"("SerialResponseEvent"=w1074, "String in"=w1077) -> ("String out"=w1075:string)  [unwired: 9 in]
                      }
                      frame True {
                        n376 = call "ProcessSerialData.vi"("SerialResponseEvent"=w1078, "String in"=w1079) -> ("String out"=w1080:string)  [unwired: 9 in]
                      }
                    }
                    n377 = Bundle By Name(cluster=w1072, "String"=w1069, "TCP"=w1066) -> (w1070:T1)
                  }
                }
              }
              event "I33 3": Value Change {
                n378 = event-data() -> ()  [unwired: 1 in, 6 out]
                n379 = Unbundle By Name(w1082) -> ("Open"=w1081:bool)
                n380 = case shown="True" w1081 {
                  tunnel: w1082 -> [w1085 w1093]
                  tunnel: [w1085 w1091] -> w1083
                  frame False {
                  }
                  frame True {
                    w1086 = "I,33,EP\n"
                    n381 = Unbundle By Name(w1093) -> ("String"=w1092:string, "PrinterResponse"=w1089:refnum<user-event>, "TCP"=w1087:refnum<k5>)
                    n382 = Empty String/Path?(string/path=w1086) -> (empty?=w1088:bool)
                    n383 = case shown="True" w1088 {
                      tunnel: w1092 -> [w1097 w1100]
                      tunnel: [w1096 w1101] -> w1090
                      tunnel: w1089 -> [w1095 w1099]
                      tunnel: w1086 -> [w1094 _]
                      frame False {
                        n384 = Concatenate Strings(w1097, w1094) -> (w1098:string)
                        n385 = call "ProcessSerialData.vi"("SerialResponseEvent"=w1095, "String in"=w1098) -> ("String out"=w1096:string)  [unwired: 9 in]
                      }
                      frame True {
                        n386 = call "ProcessSerialData.vi"("SerialResponseEvent"=w1099, "String in"=w1100) -> ("String out"=w1101:string)  [unwired: 9 in]
                      }
                    }
                    n387 = Bundle By Name(cluster=w1093, "String"=w1090, "TCP"=w1087) -> (w1091:T1)
                  }
                }
              }
              event "C33": Value Change {
                n388 = event-data() -> ()  [unwired: 1 in, 6 out]
                n389 = Unbundle By Name(w1103) -> ("Open"=w1102:bool)
                n390 = case shown="True" w1102 {
                  tunnel: w1103 -> [w1106 w1114]
                  tunnel: [w1106 w1112] -> w1104
                  frame False {
                  }
                  frame True {
                    w1107 = "C,33,0\n"
                    n391 = Unbundle By Name(w1114) -> ("String"=w1113:string, "PrinterResponse"=w1110:refnum<user-event>, "TCP"=w1108:refnum<k5>)
                    n392 = Empty String/Path?(string/path=w1107) -> (empty?=w1109:bool)
                    n393 = case shown="True" w1109 {
                      tunnel: w1113 -> [w1118 w1121]
                      tunnel: [w1117 w1122] -> w1111
                      tunnel: w1110 -> [w1116 w1120]
                      tunnel: w1107 -> [w1115 _]
                      frame False {
                        n394 = Concatenate Strings(w1118, w1115) -> (w1119:string)
                        n395 = call "ProcessSerialData.vi"("SerialResponseEvent"=w1116, "String in"=w1119) -> ("String out"=w1117:string)  [unwired: 9 in]
                      }
                      frame True {
                        n396 = call "ProcessSerialData.vi"("SerialResponseEvent"=w1120, "String in"=w1121) -> ("String out"=w1122:string)  [unwired: 9 in]
                      }
                    }
                    n397 = Bundle By Name(cluster=w1114, "String"=w1111, "TCP"=w1108) -> (w1112:T1)
                  }
                }
              }
            }
          }
          frame "Error Handler" {
            n398 = call <vilib>:"General Error Handler.vi"("error in (no error)"=w1124) -> ()  [unwired: 10 in, 5 out]
          }
          frame "UpdateSettings" {
            n399 = case shown="\"TCP\"" w1126 {
              tunnel: w1131 -> [_ w1135 w1143]
              tunnel: w1130 -> [w1133 w1136 w1144]
              tunnel: [w1133 w1137 w1145] -> w1129
              tunnel: w1128 -> [w1132 w1138 w1146]
              tunnel: [w1132 w1138 w1141] -> w1127
              frame "False", Default {
              }
              frame "Configuration" {
                n400 = Variant To Data(error in=w1136, type="placeholder", Variant=w1135) -> (error out=w1137:errorcluster)  [unwired: 1 out]
              }
              frame "TCP" {
                w1142 = refnum<k5> refnum  # TCP
                n401 = Variant To Data(error in=w1144, type=w1142, Variant=w1143) -> (data=w1140:refnum<k5>, error out=w1145:errorcluster)
                n402 = Bundle By Name(cluster=w1146, "TCP"=w1140, "Open"=TRUE) -> (w1141:T1)
              }
            }
          }
          frame "Macro: Exit" {
            n403 = call <vilib>:"Add States to Queue using MultiLine String (no vData input).vi"("queue in"=w1150, "states in"="Quit", "error in"=w1148) -> ("error out"=w1147:errorcluster)  [unwired: 10 in, 2 out]
          }
          frame "Quit" {
          }
        }
      }
    }
    frame Disabled {
      n404 = while {
        tunnel: w1155 -> [w1163]
        shift-right: [w1167] -> _
        shift-left: w1157 -> [w1169]
        shift-right: [w1164] -> _
        shift-left: w1156 -> [w1165]
        stop <- w1170 stop-if-true
        n405 = call <vilib>:"Get Next Queued State with vData.vi"("queue in"=w1163, "error in (no error)"=w1169) -> ("vData out"=w1166:variant, "queue out"=w1162:refnum<queue>, "Next State"=w1161:string, "queued msg"=w1158:string, "error out"=w1168:errorcluster)  [unwired: 7 in, 2 out]
        n406 = call <vilib>:"Parse State Queue__JKI_lib_State_Machine.vi"("State Queue"=w1161) -> ("Current State"=w1160:string, "Arguments"=w1159:string)  [unwired: 12 in, 1 out]
        n407 = case shown="\"\", \"EventHandler\", \"Idle\"" w1160 {
          tunnel: [_ _ _ _ _ _ TRUE] -> w1170
          tunnel: w1168 -> [w1172 w1176 w1180 w1346 w1352 w1370 w1375]
          tunnel: [w1172 w1176 w1179 errorcluster {"status"=FALSE, "code"=0, "source"=""} ("error out") w1351 w1369 w1375] -> w1167
          tunnel: w1166 -> [_ _ _ _ w1353 _ _]
          tunnel: w1165 -> [w1171 w1175 w1178 w1345 w1350 w1373 w1374]
          tunnel: [w1171 w1174 w1177 w1345 w1349 w1373 w1374] -> w1164
          tunnel: w1162 -> [_ _ _ _ _ w1372 _]
          tunnel: w1159 -> [_ _ _ _ _ _ _]
          tunnel: w1158 -> [_ _ _ _ w1348 _ _]
          frame Default {
          }
          frame "Initialize" {
            n408 = Bundle By Name(cluster=w1175, "Open"=FALSE) -> (w1174:T1)
          }
          frame "", "EventHandler", "Idle" {
            n409 = event shown="[1] \"A4\": Value Change" {
              selector: _ -> [_ _ _ _ _ _ _ _ _]
              dyn-events: _ -> [_ _ _ _ _ _ _ _ _]
              timeout: 1 -> [_ _ _ _ _ _ _ _ _]
              tunnel: w1178 -> [w1183 w1202 w1220 w1238 w1256 w1274 w1292 w1310 w1328]
              tunnel: w1180 -> [w1185 w1204 w1222 w1240 w1258 w1276 w1294 w1312 w1330]
              tunnel: [w1185 w1204 w1222 w1240 w1258 w1276 w1294 w1312 w1330] -> w1179
              tunnel: [w1184 w1203 w1221 w1239 w1257 w1275 w1293 w1311 w1329] -> w1177
              event Timeout {
                n410 = event-data() -> ()  [unwired: 1 in, 3 out]
                n411 = Unbundle By Name(w1183) -> ("Open"=w1182:bool)
                n412 = case shown="True" w1182 {
                  tunnel: w1183 -> [w1186 w1194]
                  tunnel: [w1186 w1192] -> w1184
                  frame False {
                  }
                  frame True {
                    n413 = Unbundle By Name(w1194) -> ("String"=w1193:string, "PrinterResponse"=w1190:refnum<user-event>, "TCP"=w1189:refnum<k5>)
                    n414 = TCP Read(connection ID=w1189) -> (data out=w1188:string)  [unwired: 4 in, 2 out]
                    n415 = Empty String/Path?(string/path=w1188) -> (empty?=w1187:bool)
                    n416 = case shown="True" w1187 {
                      tunnel: w1193 -> [w1198 w1200]
                      tunnel: [w1197 w1200] -> w1191
                      tunnel: w1190 -> [w1196 _]
                      tunnel: w1188 -> [w1195 _]
                      frame False {
                        n417 = Concatenate Strings(w1198, w1195) -> (w1199:string)
                        n418 = call "ProcessSerialData.vi"("SerialResponseEvent"=w1196, "String in"=w1199) -> ("String out"=w1197:string)  [unwired: 9 in]
                      }
                      frame True {
                      }
                    }
                    n419 = Bundle By Name(cluster=w1194, "String"=w1191) -> (w1192:T1)
                  }
                }
              }
              event "A4": Value Change {
                n420 = event-data() -> ()  [unwired: 1 in, 6 out]
                n421 = Unbundle By Name(w1202) -> ("Open"=w1201:bool)
                n422 = case shown="True" w1201 {
                  tunnel: w1202 -> [w1205 w1212]
                  tunnel: [w1205 w1210] -> w1203
                  frame False {
                  }
                  frame True {
                    w1206 = "A,44,P,V,P,PH4_Temp_Read\n"
                    n423 = Unbundle By Name(w1212) -> ("String"=w1211:string, "PrinterResponse"=w1208:refnum<user-event>)
                    n424 = Empty String/Path?(string/path=w1206) -> (empty?=w1207:bool)
                    n425 = case shown="False" w1207 {
                      tunnel: w1211 -> [w1216 w1218]
                      tunnel: [w1215 w1218] -> w1209
                      tunnel: w1208 -> [w1214 _]
                      tunnel: w1206 -> [w1213 _]
                      frame False {
                        n426 = Concatenate Strings(w1216, w1213) -> (w1217:string)
                        n427 = call "ProcessSerialData.vi"("SerialResponseEvent"=w1214, "String in"=w1217) -> ("String out"=w1215:string)  [unwired: 9 in]
                      }
                      frame True {
                      }
                    }
                    n428 = Bundle By Name(cluster=w1212, "String"=w1209) -> (w1210:T1)
                  }
                }
              }
              event "C4": Value Change {
                n429 = event-data() -> ()  [unwired: 1 in, 6 out]
                n430 = Unbundle By Name(w1220) -> ("Open"=w1219:bool)
                n431 = case shown="True" w1219 {
                  tunnel: w1220 -> [w1223 w1230]
                  tunnel: [w1223 w1228] -> w1221
                  frame False {
                  }
                  frame True {
                    w1224 = "C,44,0,40\n"
                    n432 = Unbundle By Name(w1230) -> ("String"=w1229:string, "PrinterResponse"=w1226:refnum<user-event>)
                    n433 = Empty String/Path?(string/path=w1224) -> (empty?=w1225:bool)
                    n434 = case shown="False" w1225 {
                      tunnel: w1229 -> [w1234 w1236]
                      tunnel: [w1233 w1236] -> w1227
                      tunnel: w1226 -> [w1232 _]
                      tunnel: w1224 -> [w1231 _]
                      frame False {
                        n435 = Concatenate Strings(w1234, w1231) -> (w1235:string)
                        n436 = call "ProcessSerialData.vi"("SerialResponseEvent"=w1232, "String in"=w1235) -> ("String out"=w1233:string)  [unwired: 9 in]
                      }
                      frame True {
                      }
                    }
                    n437 = Bundle By Name(cluster=w1230, "String"=w1227) -> (w1228:T1)
                  }
                }
              }
              event "A3": Value Change {
                n438 = event-data() -> ()  [unwired: 1 in, 6 out]
                n439 = Unbundle By Name(w1238) -> ("Open"=w1237:bool)
                n440 = case shown="True" w1237 {
                  tunnel: w1238 -> [w1241 w1248]
                  tunnel: [w1241 w1246] -> w1239
                  frame False {
                  }
                  frame True {
                    w1242 = "A,33,P,V,P,PH3_Temp_Read\n"
                    n441 = Unbundle By Name(w1248) -> ("String"=w1247:string, "PrinterResponse"=w1244:refnum<user-event>)
                    n442 = Empty String/Path?(string/path=w1242) -> (empty?=w1243:bool)
                    n443 = case shown="False" w1243 {
                      tunnel: w1247 -> [w1252 w1254]
                      tunnel: [w1251 w1254] -> w1245
                      tunnel: w1244 -> [w1250 _]
                      tunnel: w1242 -> [w1249 _]
                      frame False {
                        n444 = Concatenate Strings(w1252, w1249) -> (w1253:string)
                        n445 = call "ProcessSerialData.vi"("SerialResponseEvent"=w1250, "String in"=w1253) -> ("String out"=w1251:string)  [unwired: 9 in]
                      }
                      frame True {
                      }
                    }
                    n446 = Bundle By Name(cluster=w1248, "String"=w1245) -> (w1246:T1)
                  }
                }
              }
              event "C3": Value Change {
                n447 = event-data() -> ()  [unwired: 1 in, 6 out]
                n448 = Unbundle By Name(w1256) -> ("Open"=w1255:bool)
                n449 = case shown="True" w1255 {
                  tunnel: w1256 -> [w1259 w1266]
                  tunnel: [w1259 w1264] -> w1257
                  frame False {
                  }
                  frame True {
                    w1260 = "C,33,0,30\n"
                    n450 = Unbundle By Name(w1266) -> ("String"=w1265:string, "PrinterResponse"=w1262:refnum<user-event>)
                    n451 = Empty String/Path?(string/path=w1260) -> (empty?=w1261:bool)
                    n452 = case shown="False" w1261 {
                      tunnel: w1265 -> [w1270 w1272]
                      tunnel: [w1269 w1272] -> w1263
                      tunnel: w1262 -> [w1268 _]
                      tunnel: w1260 -> [w1267 _]
                      frame False {
                        n453 = Concatenate Strings(w1270, w1267) -> (w1271:string)
                        n454 = call "ProcessSerialData.vi"("SerialResponseEvent"=w1268, "String in"=w1271) -> ("String out"=w1269:string)  [unwired: 9 in]
                      }
                      frame True {
                      }
                    }
                    n455 = Bundle By Name(cluster=w1266, "String"=w1263) -> (w1264:T1)
                  }
                }
              }
              event "A2": Value Change {
                n456 = event-data() -> ()  [unwired: 1 in, 6 out]
                n457 = Unbundle By Name(w1274) -> ("Open"=w1273:bool)
                n458 = case shown="True" w1273 {
                  tunnel: w1274 -> [w1277 w1284]
                  tunnel: [w1277 w1282] -> w1275
                  frame False {
                  }
                  frame True {
                    w1278 = "A,22,P,V,P,PH2_Temp_Read\n"
                    n459 = Unbundle By Name(w1284) -> ("String"=w1283:string, "PrinterResponse"=w1280:refnum<user-event>)
                    n460 = Empty String/Path?(string/path=w1278) -> (empty?=w1279:bool)
                    n461 = case shown="False" w1279 {
                      tunnel: w1283 -> [w1288 w1290]
                      tunnel: [w1287 w1290] -> w1281
                      tunnel: w1280 -> [w1286 _]
                      tunnel: w1278 -> [w1285 _]
                      frame False {
                        n462 = Concatenate Strings(w1288, w1285) -> (w1289:string)
                        n463 = call "ProcessSerialData.vi"("SerialResponseEvent"=w1286, "String in"=w1289) -> ("String out"=w1287:string)  [unwired: 9 in]
                      }
                      frame True {
                      }
                    }
                    n464 = Bundle By Name(cluster=w1284, "String"=w1281) -> (w1282:T1)
                  }
                }
              }
              event "C2": Value Change {
                n465 = event-data() -> ()  [unwired: 1 in, 6 out]
                n466 = Unbundle By Name(w1292) -> ("Open"=w1291:bool)
                n467 = case shown="True" w1291 {
                  tunnel: w1292 -> [w1295 w1302]
                  tunnel: [w1295 w1300] -> w1293
                  frame False {
                  }
                  frame True {
                    w1296 = "C,22,0,20\n"
                    n468 = Unbundle By Name(w1302) -> ("String"=w1301:string, "PrinterResponse"=w1298:refnum<user-event>)
                    n469 = Empty String/Path?(string/path=w1296) -> (empty?=w1297:bool)
                    n470 = case shown="False" w1297 {
                      tunnel: w1301 -> [w1306 w1308]
                      tunnel: [w1305 w1308] -> w1299
                      tunnel: w1298 -> [w1304 _]
                      tunnel: w1296 -> [w1303 _]
                      frame False {
                        n471 = Concatenate Strings(w1306, w1303) -> (w1307:string)
                        n472 = call "ProcessSerialData.vi"("SerialResponseEvent"=w1304, "String in"=w1307) -> ("String out"=w1305:string)  [unwired: 9 in]
                      }
                      frame True {
                      }
                    }
                    n473 = Bundle By Name(cluster=w1302, "String"=w1299) -> (w1300:T1)
                  }
                }
              }
              event "A1": Value Change {
                n474 = event-data() -> ()  [unwired: 1 in, 6 out]
                n475 = Unbundle By Name(w1310) -> ("Open"=w1309:bool)
                n476 = case shown="True" w1309 {
                  tunnel: w1310 -> [w1313 w1320]
                  tunnel: [w1313 w1318] -> w1311
                  frame False {
                  }
                  frame True {
                    w1314 = "A,11,P,V,P,PH1_Temp_Read\n"
                    n477 = Unbundle By Name(w1320) -> ("String"=w1319:string, "PrinterResponse"=w1316:refnum<user-event>)
                    n478 = Empty String/Path?(string/path=w1314) -> (empty?=w1315:bool)
                    n479 = case shown="False" w1315 {
                      tunnel: w1319 -> [w1324 w1326]
                      tunnel: [w1323 w1326] -> w1317
                      tunnel: w1316 -> [w1322 _]
                      tunnel: w1314 -> [w1321 _]
                      frame False {
                        n480 = Concatenate Strings(w1324, w1321) -> (w1325:string)
                        n481 = call "ProcessSerialData.vi"("SerialResponseEvent"=w1322, "String in"=w1325) -> ("String out"=w1323:string)  [unwired: 9 in]
                      }
                      frame True {
                      }
                    }
                    n482 = Bundle By Name(cluster=w1320, "String"=w1317) -> (w1318:T1)
                  }
                }
              }
              event "C1": Value Change {
                n483 = event-data() -> ()  [unwired: 1 in, 6 out]
                n484 = Unbundle By Name(w1328) -> ("Open"=w1327:bool)
                n485 = case shown="True" w1327 {
                  tunnel: w1328 -> [w1331 w1338]
                  tunnel: [w1331 w1336] -> w1329
                  frame False {
                  }
                  frame True {
                    w1332 = "C,11,0,10\n"
                    n486 = Unbundle By Name(w1338) -> ("String"=w1337:string, "PrinterResponse"=w1334:refnum<user-event>)
                    n487 = Empty String/Path?(string/path=w1332) -> (empty?=w1333:bool)
                    n488 = case shown="False" w1333 {
                      tunnel: w1337 -> [w1342 w1344]
                      tunnel: [w1341 w1344] -> w1335
                      tunnel: w1334 -> [w1340 _]
                      tunnel: w1332 -> [w1339 _]
                      frame False {
                        n489 = Concatenate Strings(w1342, w1339) -> (w1343:string)
                        n490 = call "ProcessSerialData.vi"("SerialResponseEvent"=w1340, "String in"=w1343) -> ("String out"=w1341:string)  [unwired: 9 in]
                      }
                      frame True {
                      }
                    }
                    n491 = Bundle By Name(cluster=w1338, "String"=w1335) -> (w1336:T1)
                  }
                }
              }
            }
          }
          frame "Error Handler" {
            n492 = call <vilib>:"General Error Handler.vi"("error in (no error)"=w1346) -> ()  [unwired: 10 in, 5 out]
          }
          frame "UpdateSettings" {
            n493 = case shown="\"TCP\"" w1348 {
              tunnel: w1353 -> [_ w1357 w1365]
              tunnel: w1352 -> [w1355 w1358 w1366]
              tunnel: [w1355 w1359 w1367] -> w1351
              tunnel: w1350 -> [w1354 w1360 w1368]
              tunnel: [w1354 w1360 w1363] -> w1349
              frame "False", Default {
              }
              frame "Configuration" {
                n494 = Variant To Data(error in=w1358, type="placeholder", Variant=w1357) -> (error out=w1359:errorcluster)  [unwired: 1 out]
              }
              frame "TCP" {
                w1364 = refnum<k5> refnum  # TCP
                n495 = Variant To Data(error in=w1366, type=w1364, Variant=w1365) -> (data=w1362:refnum<k5>, error out=w1367:errorcluster)
                n496 = Bundle By Name(cluster=w1368, "TCP"=w1362, "Open"=TRUE) -> (w1363:T1)
              }
            }
          }
          frame "Macro: Exit" {
            n497 = call <vilib>:"Add States to Queue using MultiLine String (no vData input).vi"("queue in"=w1372, "states in"="Quit", "error in"=w1370) -> ("error out"=w1369:errorcluster)  [unwired: 10 in, 2 out]
          }
          frame "Quit" {
          }
        }
      }
    }
  }
  "GIS Printer out" <- "GIS Printer in"
